vi "运维调试_总磷.vi"() -> ()   [LabVIEW 2016, in "斯坦道总磷.lvlib"]
uses:
  <vilib>/Utility/miscctls.llb/LVPointTypeDef.ctl
  <vilib>/Utility/config.llb/NI_LVConfig.lvlib
  <vilib>/ptbypt/NI_PtbyPt.lvlib
panel:
  in  "远程标样校准":enum16{"标液1", "标液2", "标液3", "标液4"}(ring)
  in  "远程校准量程":enum16{"低量程", "高量程"}(ring)
  out "固件版本号":string
  in  "定时设置":cluster{"启动":bool, "控制命令":T1, "测量参数":T2}(xcontrol)
  out "模块版本号":string
  out "单位:":T3(ring)
  out "运行状态":T4 {"数据时间:" format="%<%y/%m/%d %H:%M:%S>T"; "仪器时间:" format="%<%y/%m/%d %H:%M:%S>T"}
  in  "校准按钮":T5
  out "温度2":sgl
  out "温度1":sgl
  out "ADC":sgl
  out "F3":sgl format="%#.6f"
  out "F2":sgl format="%#.6f"
  out "F1":sgl format="%#.6f"
  out "F0":sgl format="%#.6f"
  out "二级权限":bool
  out "一级权限":bool
  out "输入密码":u32
  out "权限锁":bool
  in  "流程固件":bool
  in  "仪器参数设置":bool
  in  "量程参数读取":T6
  in  "模块启用":bool
  in  "串口设置":bool
  in  "公式一键写入":bool
  in  "流程路径":path=path "C:/Users/STD/Documents/斯坦道流程文件/流程.xml"
  in  "曲线模型":cluster{"X^2":dbl, "X":dbl, "B":dbl, "r^2":dbl}(xcontrol)
  out "字符串":string
  in  "质控参数设置":bool
  in  "数组":string[](array[string])
  in  "量程切换阈值写入":bool
  in  "量程切换阈值读取":bool
  in  "参数下拉列表":enum16{"总磷", "总氮"}(ring)
  in  "量程下拉列表":enum16{"低量程", "高量程"}(ring)
  in  "测量模式下拉列表":enum16{"水样测量", "零点核查", "跨度核查", "标样核查", "加标回收"}(ring)
  in  "公式":cluster{"X^2":dbl, "X":dbl, "b":dbl}
  in  "写公式":bool
  in  "读公式":bool
  in  "返回":bool
  in  "设置":bool
  out "集成报警信息":string
  in  "停止":bool
  in  "手动启动":bool
  in  "单步测试":bool
  out "多列列表框":i32(listbox)
  # "参数设置"
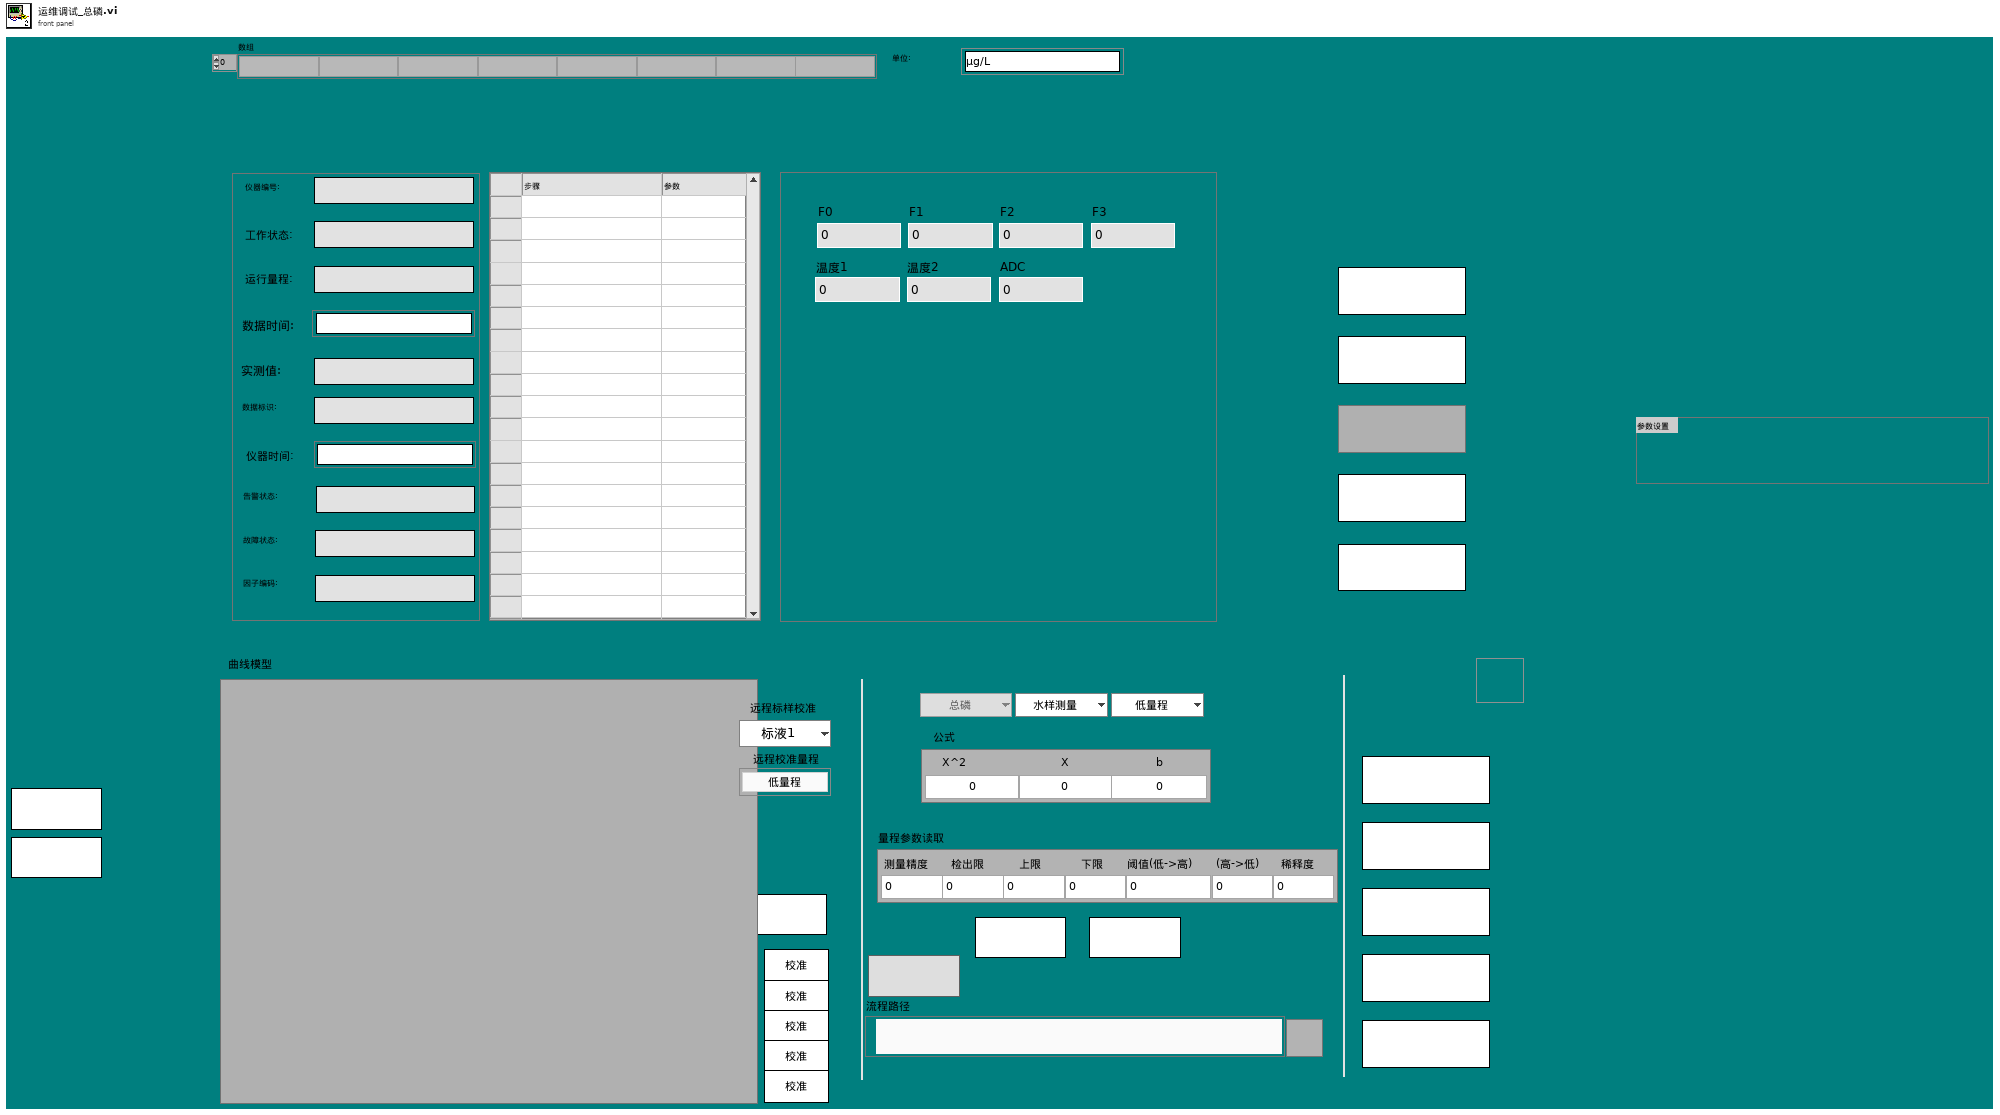
[diagram p1: front panel]
types:
  T1 = typedef "定时设置.xctl/国标控制命令.ctl" = enum16{"启动测量", "标样核查", "零点核查", "跨度核查", "空白测试", "平行样测试", "加标回收", "空白校准", "标样校准", "初始化（清洗）", "停止测试", "仪器重启", "校时", "模式设置", "测量间隔设置"}
  T2 = typedef "定时设置.xctl/测量参数.ctl" = u16
  T3 = enum16{"μg/L", "mg/L", "ppm", "mg/m3", "cm", "ppb", "μg/m3", "%", "nmol/mol", "μmol/mol", "MPN/L", "MPN/100ml", "ng/m3", "NTU", "无量纲", "mS/cm", "μS/cm", "℃", "mV", "cells/L"}
  T4 = cluster{"仪器编号:":string, "工作状态:":string, "运行量程: ":string, "数据时间:":timestamp, "实测值:":string, "数据标识: ":string, "仪器时间:":timestamp, "告警状态: ":string, "故障状态:  ":string, "因子编码:":string}
  T5 = cluster{"校准1":bool, "校准2":bool, "校准3":bool, "校准4":bool, "校准5":bool}
  T6 = cluster{"测量精度":dbl, "检出限":dbl, "上限":dbl, "下限":dbl, "阈值(低->高)":dbl, "(高->低)":dbl, "稀释度":dbl}
  T7 = cluster{"时间源选择":enum16{"系统时间源", "仪器时间源"}, "外部时间源":timestamp}
  T8 = cluster{"系统时间":timestamp, "工作状态":enum16{"空闲", "水样测试", "标样核查", "零点核查", "跨度核查", "空白测试", "平行样测试", "加标回收", "空白校准", "标样校准", "初始化（清洗）"}, "测量模式":enum16{"待机", "连续模式", "周期模式", "定点模式", "受控模式", "手动模式"}, "告警代码":u16, "故障代码":u16, "日志代码":u16, "软件版本":u16, "F0":sgl, "F1":sgl, "F2":sgl, "F3":sgl, "T":sgl, "H":sgl, "id":u16, "flowid":u16, "量程":u16, "总磷控温温度1":sgl, "营养盐控温温度2":sgl, "ADC":sgl}
  T9 = enum32{"Bad", "Idle", "Run top level", "Running"}
  T10 = enum16{"空闲", "水样测试", "标样核查", "零点核查", "跨度核查", "空白测试", "平行样测试", "加标回收", "空白校准", "标样校准", "初始化（清洗）"}
  T11 = typedef "LVPointTypeDef.ctl" = cluster{"Horizontal":i16, "Vertical":i16}
  T12 = cluster{"因子编码":u32, "单位":u16, "标样参考值":sgl, "水样数据时间":timestamp, "水样实测值":sgl, "水样数据标识":string, "标样数据时间":timestamp, "标样实测值":sgl, "标样数据标识":string, "空白数据时间":timestamp, "空白实测值":sgl, "空白数据标识":string, "零点核查数据时间":timestamp, "零点核查实测值":sgl, "零点核查数据标识":string, "跨度核查数据时间":timestamp, "跨度核查实测值":sgl, "跨度核查数据标识":string, "加标回收数据时间":timestamp, "加标回收实测值":sgl, "加标回收数据标识":string, "平行样数据时间":timestamp, "平行样实测值":sgl, "平行样数据标识":string, "F0":sgl, "F1":sgl, "F2":sgl, "F3":sgl, "F4":sgl, "F5":sgl, "F6":sgl, "F7":sgl, "温度":sgl, "湿度":sgl, "X值":sgl, "fidrange":u16}
  T13 = enum16{"待机", "连续模式", "周期模式", "定点模式", "受控模式", "手动模式"}
  T14 = cluster{"Major":u16, "Minor":u16, "Fix":u16, "Build":u16}
  T15 = typedef "NI_LVConfig.lvlib/Config Data RefNum.ctl" = refnum<k1>
  T16 = enum8{"Enabled", "Disabled", "Disabled and Grayed Out"}
  T17 = cluster{"运行模式":enum16{"维护模式", "常规模式", "应急模式", "质控模式"}, "质控频次":enum16{"关闭", "每天", "星期一", "星期二", "星期三", "星期四", "星期五", "星期六", "星期日"}, "空白核查时间":u16, "跨度核查时间":u16, "24H周期设置":bool[]}
  T18 = cluster{"时间标识":timestamp, "设备":string, "日志信息":string, "备注":string}
  T19 = cluster{"参数":string, "报警内容":string, "报警分析":string}
  T20 = cluster{"启动模式":enum16{"跨度核查", "水样测量", "空白核查", "标样核查", "加标回收"}, "启动参数":u16, "量程":enum16{"低量程", "高量程"}}
  T21 = cluster{"时间标识":timestamp, "设备":string, "日志信息":string, "流程参数":string}
  T22 = typedef "LVRowAndColumnUnsignedTypeDef.ctl" = cluster{"Row":u32, "Column":u32}
  T23 = cluster{"参数下拉列表":enum16{"总磷", "总氮"}, "测量模式下拉列表":enum16{"水样测量", "零点核查", "跨度核查", "标样核查", "加标回收"}, "量程下拉列表":enum16{"低量程", "高量程"}}
  T24 = cluster{"站号":u16, "量程切换":enum32{"H", "L", "AUTO"}, "控制命令":enum16{"启动测量", "标样核查", "零点核查", "跨度核查", "空白测试", "平行样测试", "加标回收", "空白校准", "标样校准", "初始化（清洗）", "停止测试", "仪器重启", "校时", "模式设置", "测量间隔设置"}, "模式设置":enum16{"待机", "连续模式", "周期模式", "定点模式", "受控模式", "手动模式"}, "测量间隔":u16}
  T25 = cluster{"水样测试量程模式":enum16{"H", "L", "AUTO"}, "空白核查量程模式":enum16{"H", "L", "AUTO"}, "跨度核查量程模式":enum16{"H", "L", "AUTO"}, "加标回收量程模式":enum16{"H", "L", "AUTO"}}
  T26 = cluster{"总磷跨度值":dbl, "总磷零点标准液浓度":dbl, "总磷跨度标准液浓度":dbl, "总磷标准液标准浓度":dbl}
  T27 = cluster{"确定":bool, "总磷跨度值":dbl, "总磷零点标准液浓度":dbl, "总磷跨度标准液浓度":dbl, "总磷标准液标准浓度":dbl}
  T28 = cluster{"测量量程":dbl, "测量精度":dbl, "测量间隔":dbl, "消解温度":dbl, "消解时长":dbl, "空白校准时间":timestamp, "曲线截距":dbl, "曲线斜率":dbl, "测量检出限":dbl, "测量信号值":dbl, "线性相关系数":dbl, "二次多项式系数":dbl, "标样校准时间":timestamp, "稀释倍数":dbl, "三项式系数":dbl, "空白标定系数":dbl, "量程系数":dbl, "F0/ORPA":dbl, "F1/ORPB":dbl, "F2/ORPK":dbl, "F3":dbl, "F4":dbl, "F5":dbl, "F6":dbl, "F7":dbl, "X0/滴定数":dbl, "量程":dbl}
  T29 = cluster{"确定":bool, "测量量程":dbl, "测量精度":dbl, "测量间隔":dbl, "消解温度":dbl, "消解时长":dbl, "空白校准时间":timestamp, "曲线截距":dbl, "曲线斜率":dbl, "测量检出限":dbl, "测量信号值":dbl, "线性相关系数":dbl, "二次多项式系数":dbl, "标样校准时间":timestamp, "稀释倍数":dbl, "三项式系数":dbl, "空白标定系数":dbl, "量程系数":dbl, "F0/ORPA":dbl, "F1/ORPB":dbl, "F2/ORPK":dbl, "F3":dbl, "F4":dbl, "F5":dbl, "F6":dbl, "F7":dbl, "X0/滴定数":dbl, "量程":dbl}
  T30 = cluster{"标液浓度1":dbl, "标液浓度2":dbl, "标液浓度3":dbl, "标液浓度4":dbl, "标液浓度5":dbl}
  T31 = cluster{"测量精度":u16, "检出限":dbl, "上限":dbl, "下限":dbl, "阈值（低->高）":dbl, "阈值（高->低）":dbl, "稀释度":dbl}
  T32 = enum16{"Left Button", "Center Button", "Right Button", "Window Close"}
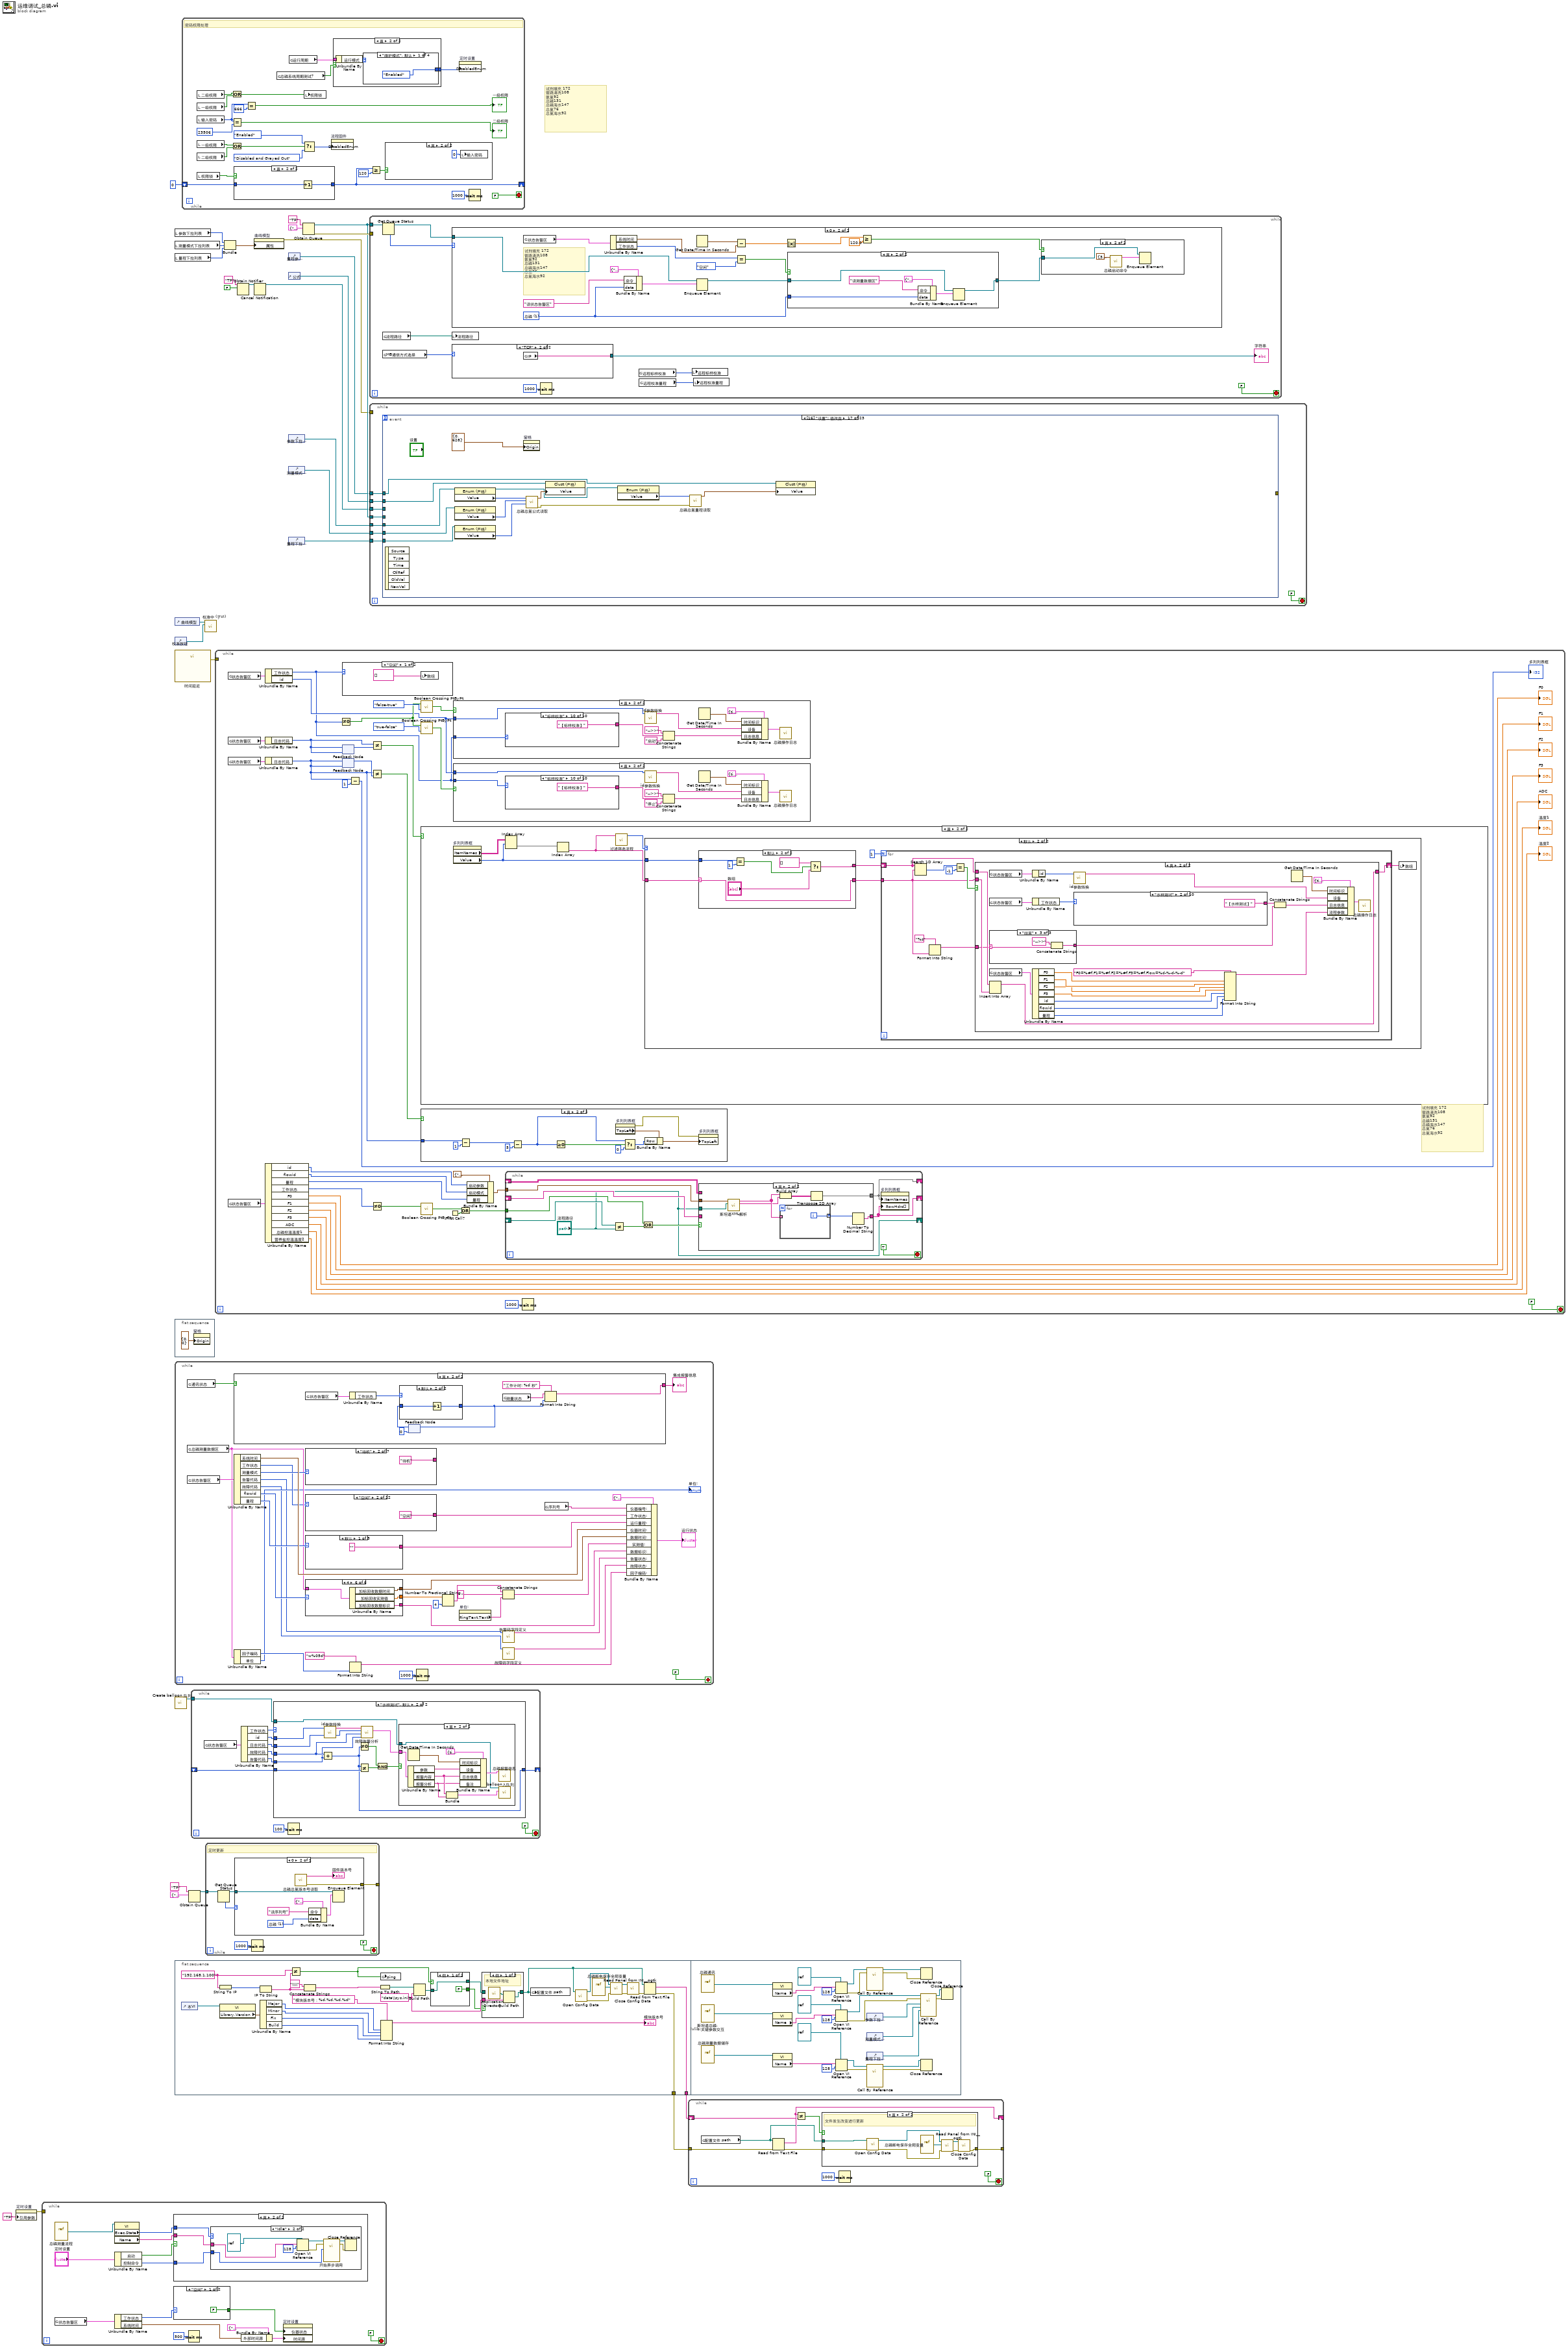
[diagram p0: block diagram]
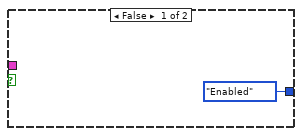
[diagram p5: hidden frame]
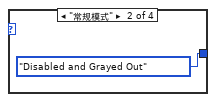
[diagram p6: hidden frame]
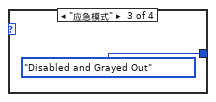
[diagram p7: hidden frame]
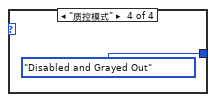
[diagram p8: hidden frame]
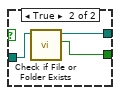
[diagram p11: hidden frame]
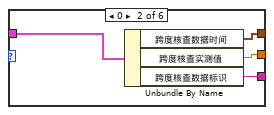
[diagram p15: hidden frame]
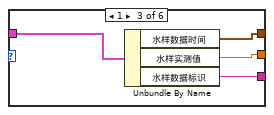
[diagram p16: hidden frame]
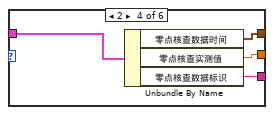
[diagram p17: hidden frame]
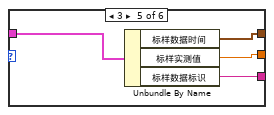
[diagram p18: hidden frame]
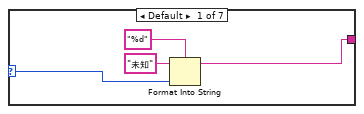
[diagram p19: hidden frame]
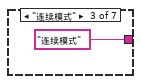
[diagram p20: hidden frame]
diagram:
  # "试剂填充 172 \n管路清洗108\n氨氮92\n总磷131\n总磷海水147\n总氮76\n总氮海水92"
  n1 = property on="定时设置" class="定时设置 (严格)"("引用参数"="TP") -> (error out=w1:errorcluster)  [unwired: 2 in, 1 out]
  n2 = while {
    tunnel: w1 -> [_]
    stop <- FALSE stop-if-true
    n3 = vi-ref "总磷测量流程.vi"() -> (w42:refnum<vi>)
    n4 = global read "VAR总磷全局变量.vi" "状态告警区"() -> (w36:T8)
    n5 = property class="VI"(reference=w42) -> ("Exec.State"=w40:T9, "Name"=w41:string)  [unwired: 1 in, 2 out]
    n6 = Unbundle By Name("定时设置") -> ("启动"=w37:bool, "控制命令"=w38:T1)
    n7 = Unbundle By Name(w36) -> ("工作状态"=w35:T10, "系统时间"=w32:timestamp)
    n8 = case shown="真" w37 {
      tunnel: w41 -> [_ w49]
      tunnel: w38 -> [_ w48]
      tunnel: w40 -> [_ w47]
      frame False {
      }
      frame True {
        n9 = case shown="\"Idle\"" w47 {
          tunnel: w49 -> [_ w53]
          tunnel: w48 -> [_ w51]
          frame "Bad", Default {
          }
          frame "Idle" {
            n10 = Open VI Reference(type specifier VI Refnum (for type only)=refnum<vi> refnum, vi path=w53, options=128 ("选项")) -> (vi reference=w54:refnum<vi>, error out=w55:errorcluster)  [unwired: 3 in]
            n11 = call-by-ref "开始异步调用"(reference=w54, error in=w55, "控制命令"=w51) -> (reference out=w56:refnum<vi>, error out=w57:errorcluster)  [unwired: 11 in]
            n12 = Close Reference(reference=w56, error in (no error)=w57) -> ()  [unwired: 1 out]
          }
        }
      }
    }
    n13 = case shown="\"空闲\"" w35 {
      tunnel: [FALSE TRUE] -> w34
      frame "空闲" {
      }
      frame "水样测试", Default {
      }
    }
    n14 = Wait (ms)(milliseconds to wait=u32 500 ("等待时间（毫秒）")) -> ()  [unwired: 1 out]
    n15 = Bundle By Name(cluster=T7 {"时间源选择"=enum."仪器时间源", "外部时间源"=timestamp(0 s since 1904-01-01)} ("时间源"), "外部时间源"=w32) -> (w31:T7)
    n16 = property on="定时设置" class="定时设置 (严格)"("仪器状态"=w34, "时间源"=w31) -> ()  [unwired: 2 in, 2 out]
  }
  n17 = local read "参数下拉列表"() -> (w11:enum16{"总磷", "总氮"})
  n18 = local read "测量模式下拉列表"() -> (w10:enum16{"水样测量", "零点核查", "跨度核查", "标样核查", "加标回收"})
  n19 = local read "量程下拉列表"() -> (w9:enum16{"低量程", "高量程"})
  n20 = control-ref of="曲线模型"() -> (w5:refnum<vi>)
  n21 = control-ref of="校准按钮"() -> (w6:refnum<vi>)
  n22 = call "时间延迟"() -> ("error out"=w22:errorcluster)  [unwired: 11 in]
  n23 = flat-sequence {
    frame #0 {
      n24 = property on="窗格" class="Pane"("Origin"=T11 {"Horizontal"=0, "Vertical"=0} ("原点")) -> ()  [unwired: 2 in, 2 out]
    }
  }
  n25 = while {
    stop <- FALSE stop-if-true
    n26 = global read "VAR总磷全局变量.vi" "通讯状态"() -> (w88:bool)
    n27 = global read "VAR总磷全局变量.vi" "总磷测量数据区"() -> (w78:T12)
    n28 = global read "VAR总磷全局变量.vi" "状态告警区"() -> (w79:T8)
    n29 = case shown="真" w88 {
      tunnel: ["通讯异常" ("集成报警信息") w141] -> w87
      frame False {
      }
      frame True {
        n30 = global read "VAR总磷全局变量.vi" "状态告警区"() -> (w147:T8)
        n31 = Unbundle By Name(w147) -> ("工作状态"=w146:T10)
        n32 = feedback #1(0) -> (w144:i32)
        n33 = case shown="默认" w146 {
          tunnel: w144 -> [_ w149]
          tunnel: [_ w148] -> w142
          frame "空闲" {
          }
          frame Default {
            n34 = Increment(x=w149) -> (x+1=w148:i32)
          }
        }
        n35 = feedback-in #1(w142) -> ()
        n36 = global read "VAR总磷全局变量.vi" "测量状态"() -> (w140:string)
        n37 = Format Into String(format string="工作计时: %d 秒" ("格式字符串"), initial string=w140, w142) -> (resulting string=w141:string)  [unwired: 1 in, 1 out]
      }
    }
    "集成报警信息" <- w87
    n38 = Unbundle By Name(w79) -> ("系统时间"=w86:timestamp, "工作状态"=w76:T10, "测量模式"=w82:T13, "告警代码"=w62:u16, "故障代码"=w60:u16, "flowid"=w75:u16, "量程"=w84:u16)
    n39 = Unbundle By Name(w78) -> ("因子编码"=w80:u32, "单位"=→"单位:":u16)
    n40 = case shown="\"待机\"" w82 {
      selector: w82 -> [w111 _ _ _ _ _ _]
      tunnel: [w112 "待机" "连续模式" "周期模式" "定点模式" "受控模式" "手动模式"] -> _
      frame Default {
        n41 = Format Into String(format string="%d" ("格式字符串"), initial string="未知" ("工作状态"), w111) -> (resulting string=w112:string)  [unwired: 1 in, 1 out]
      }
      frame "待机" {
      }
      frame "连续模式" {
      }
      frame "周期模式" {
      }
      frame "定点模式" {
      }
      frame "受控模式" {
      }
      frame "手动模式" {
      }
    }
    n42 = case shown="\"空闲\"" w76 {
      selector: w76 -> [w124 _ _ _ _ _ _ _ _ _ _ _]
      tunnel: [w125 "空闲" ("工作状态") "水样测量" ("工作状态") "标样核查" ("工作状态") "零点核查" ("工作状态") "跨度核查" ("工作状态") "空白测试" ("工作状态") "平行样测试" ("工作状态") "加标回收" ("工作状态") "空白校准" ("工作状态") "标样校准" ("工作状态") "初始化" ("工作状态")] -> w85
      frame Default {
        n43 = Format Into String(format string="%d" ("格式字符串"), initial string="未知" ("工作状态"), w124) -> (resulting string=w125:string)  [unwired: 1 in, 1 out]
      }
      frame "空闲" {
      }
      frame "水样测试" {
      }
      frame "标样核查" {
      }
      frame "零点核查" {
      }
      frame "跨度核查" {
      }
      frame "空白测试" {
      }
      frame "平行样测试" {
      }
      frame "加标回收" {
      }
      frame "空白校准" {
      }
      frame "标样校准" {
      }
      frame "初始化（清洗）" {
      }
    }
    n44 = case shown="默认" w84 {
      tunnel: ["" ("字符串") "低量程" ("字符串") "高量程" ("字符串")] -> w83
      frame Default {
      }
      frame 0 {
      }
      frame 1 {
      }
    }
    n45 = case shown="4" w75 {
      tunnel: [_ w94 w98 w102 w106 w110] -> w72
      tunnel: [_ w92 w97 w101 w105 w109] -> w68
      tunnel: [_ w91 w96 w100 w104 w108] -> w64
      tunnel: w78 -> [_ w93 w95 w99 w103 w107]
      frame Default {
      }
      frame 0 {
        n46 = Unbundle By Name(w93) -> ("跨度核查数据时间"=w94:timestamp, "跨度核查实测值"=w92:sgl, "跨度核查数据标识"=w91:string)
      }
      frame 1 {
        n47 = Unbundle By Name(w95) -> ("水样数据时间"=w98:timestamp, "水样实测值"=w97:sgl, "水样数据标识"=w96:string)
      }
      frame 2 {
        n48 = Unbundle By Name(w99) -> ("零点核查数据时间"=w102:timestamp, "零点核查实测值"=w101:sgl, "零点核查数据标识"=w100:string)
      }
      frame 3 {
        n49 = Unbundle By Name(w103) -> ("标样数据时间"=w106:timestamp, "标样实测值"=w105:sgl, "标样数据标识"=w104:string)
      }
      frame 4 {
        n50 = Unbundle By Name(w107) -> ("加标回收数据时间"=w110:timestamp, "加标回收实测值"=w109:sgl, "加标回收数据标识"=w108:string)
      }
    }
    n51 = Format Into String(format string="w%05d" ("格式字符串"), w80) -> (resulting string=w63:string)  [unwired: 2 in, 1 out]
    n52 = Wait (ms)(milliseconds to wait=u32 1000 ("等待时间（毫秒）")) -> ()  [unwired: 1 out]
    n53 = Number To Fractional String(number=w68, precision (6)=i16 4 ("精度(6)")) -> (F-format string=w70:string)  [unwired: 2 in]
    n54 = property on="单位:" class="Enum (严格)"() -> ("RingText.Text"=w66:string)  [unwired: 2 in, 2 out]
    n55 = Concatenate Strings(w70, " " ("字符串"), w66) -> (w65:string)
    n56 = call "告警码字段定义.vi"("告警代码"=w62) -> ("字符串"=w61:string)  [unwired: 8 in, 2 out]
    n57 = call "故障码字段定义.vi"("故障代码"=w60) -> ("字符串"=w59:string)  [unwired: 10 in]
    n58 = global read "VAR总磷全局变量.vi" "序列号"() -> (w77:string)
    n59 = Bundle By Name(cluster=T4 {"仪器编号:"="", "工作状态:"="", "运行量程: "="", "数据时间:"=timestamp(0 s since 1904-01-01), "实测值:"="", "数据标识: "="", "仪器时间:"=timestamp(0 s since 1904-01-01), "告警状态: "="", "故障状态:  "="", "因子编码:"=""} ("运行状态"), "仪器编号:"=w77, "工作状态:"=w85, "运行量程:"=w83, "仪器时间:"=w86, "数据时间:"=w72, "实测值:"=w65, "数据标识:"=w64, "告警状态:"=w61, "故障状态:"=w59, "因子编码:"=w63) -> (→"运行状态":T4)
  }
  n60 = call "Create balloon 队列.vi"() -> ("队列输出"=w3:refnum<queue>)  [unwired: 11 in]
  n61 = flat-sequence {
    tunnel: [w159] -> w4
    tunnel: [w158] -> w7
    frame #0 {
      w172 = "data\\sys.ini" ("名称或相对路径")
      w164 = "192.168.1.100" ("名称")
      n62 = control-ref of="本VI"() -> (w157:refnum<vi>)
      n63 = String To IP(1:w164) -> (0:w171:u32)
      n64 = property class="VI"(reference=w157) -> ("Library.Version"=w156:T14)  [unwired: 1 in, 2 out]
      n65 = IP To String(2:w171) -> (0:w168:string)  [unwired: 1 in]
      n66 = Unbundle By Name(w156) -> ("Major"=w154:u16, "Minor"=w153:u16, "Fix"=w152:u16, "Build"=w151:u16)
      n67 = Not Equal?(x=w164, y=w168) -> (x != y?=w162:bool)
      n68 = Concatenate Strings("\\\\" ("字符串"), w168) -> (w169:string)
      n69 = String To Path(string=w169) -> (path=w163:path)
      n70 = global write "VAR总磷全局变量.vi" "ping"(w162) -> ()
      n71 = Format Into String(format string="模块版本号：%d.%d.%d.%d" ("格式字符串"), w154, w153, w152, w151) -> (resulting string=→"模块版本号":string)  [unwired: 2 in, 1 out]
      n72 = Build Path(base path=w163, name or relative path=w172) -> (appended path=w167:path)
      n73 = case shown="假" w162 {
        tunnel: w167 -> [w178 w182]
        tunnel: [w178 w181] -> w166
        tunnel: [FALSE w180] -> w165
        frame False {
        }
        frame True {
          n74 = call <vilib>:"Check if File or Folder Exists.vi"("path"=w182) -> ("file or folder exists?"=w180:bool, "dup path"=w181:path)  [unwired: 8 in, 1 out]
        }
      }
      n75 = case shown="假" w165 {
        tunnel: w166 -> [_ w186]
        tunnel: [w184 w186] -> w161
        tunnel: w172 -> [w183 _]
        frame False {
          # "本地文件地址"
          n76 = call <vilib>:"Application Directory.vi"() -> ("Application Directory"=w185:path)
          n77 = Build Path(base path=w185, name or relative path=w183) -> (appended path=w184:path)
        }
        frame True {
          # "网络共享地址"
        }
      }
      n78 = global write "VAR总磷全局变量.vi" "配置文件 path"(w161) -> ()
      n79 = call <vilib>:"Open Config Data.vi"("configuration file path"=w161) -> ("error out"=w174:errorcluster, "refnum"=w177:T15)  [unwired: 8 in, 1 out]
      n80 = vi-ref "总磷断电保存全局变量.vi"() -> (w176:refnum<vi>)
      n81 = call <userlib>:"Read Panel from INI__ogtk.vi"("error in (no error)"=w174, "VI ref"=w176, "refnum"=w177) -> ("error out"=w173:errorcluster, "refnum out"=w175:T15)  [unwired: 7 in]
      n82 = call <vilib>:"Close Config Data.vi"("error in (no error)"=w173, "refnum"=w175) -> ("error out"=w160:errorcluster)  [unwired: 8 in, 1 out]
      n83 = Read from Text File(file (use dialog)=w161, error in=w160) -> (text=w158:string, error out=w159:errorcluster)  [unwired: 2 in, 2 out]
    }
    frame #1 {
      n84 = vi-ref "总磷通讯.vi"() -> (w213:refnum<vi>)
      n85 = vi-ref "斯坦道总磷.lvlib:关键参数交互.vi"() -> (w190:refnum<vi>)
      n86 = vi-ref "总磷测量数据储存.vi"() -> (w205:refnum<vi>)
      n87 = property class="VI"(reference=w213) -> ("Name"=w212:string)  [unwired: 1 in, 2 out]
      n88 = property class="VI"(reference=w190) -> ("Name"=w191:string)  [unwired: 1 in, 2 out]
      n89 = property class="VI"(reference=w205) -> ("Name"=w198:string)  [unwired: 1 in, 2 out]
      n90 = Open VI Reference(type specifier VI Refnum (for type only)=refnum<vi> refnum, vi path=w212, options=128 ("选项")) -> (vi reference=w210:refnum<vi>, error out=w208:errorcluster)  [unwired: 3 in]
      n91 = Open VI Reference(type specifier VI Refnum (for type only)=refnum<vi> refnum, vi path=w191, options=128 ("选项")) -> (vi reference=w193:refnum<vi>, error out=w195:errorcluster)  [unwired: 3 in]
      n92 = Open VI Reference(type specifier VI Refnum (for type only)=refnum<vi> refnum, vi path=w198, options=128 ("选项")) -> (vi reference=w200:refnum<vi>, error out=w202:errorcluster)  [unwired: 3 in]
      n93 = call-by-ref "?"(reference=w210, error in=w208) -> (reference out=w206:refnum<vi>, error out=w207:errorcluster)  [unwired: 12 in]
      n94 = control-ref of="参数下拉列表"() -> (w187:refnum<vi>)
      n95 = control-ref of="测量模式下拉列表"() -> (w188:refnum<vi>)
      n96 = control-ref of="量程下拉列表"() -> (w189:refnum<vi>)
      n97 = call-by-ref "?"(reference=w200, error in=w202) -> (reference out=w204:refnum<vi>, error out=w203:errorcluster)  [unwired: 12 in]
      n98 = Close Reference(reference=w206, error in (no error)=w207) -> ()  [unwired: 1 out]
      n99 = call-by-ref "?"(reference=w193, error in=w195, "量程下拉列表"=w189, "测量模式下拉列表"=w188, "测量参数"=w187) -> (reference out=w197:refnum<vi>, error out=w196:errorcluster)  [unwired: 9 in]
      n100 = Close Reference(reference=w204, error in (no error)=w203) -> ()  [unwired: 1 out]
      n101 = Close Reference(reference=w197, error in (no error)=w196) -> ()  [unwired: 1 out]
    }
  }
  n102 = while {
    shift-right: [w219] -> _
    shift-left: u32 0 ("等待时间（毫秒）") -> [w220]
    stop <- FALSE stop-if-true
    # "密码权限处理"
    n103 = local read "二级权限"() -> (w227:bool)
    n104 = local read "一级权限"() -> (w233:bool)
    n105 = local read "输入密码"() -> (w231:u32)
    n106 = local read "一级权限"() -> (w232:bool)
    n107 = local read "二级权限"() -> (w222:bool)
    n108 = local read "权限锁"() -> (w221:bool)
    n109 = Or(x=w227, y=w233) -> (x .or. y?=w228:bool)
    n110 = Equal?(x=w231, y=u32 23506) -> (x = y?=→"二级权限":bool)
    n111 = Or(x=w232, y=w222) -> (x .or. y?=w223:bool)
    n112 = case shown="真" w221 {
      tunnel: w220 -> [_ w248]
      tunnel: [_ w247] -> w219
      frame False {
      }
      frame True {
        n113 = Increment(x=w248) -> (x+1=w247:u32)
      }
    }
    n114 = Equal?(x=w231, y=u32 666) -> (x = y?=→"一级权限":bool)
    n115 = global read "总磷断电保存全局变量.vi" "总磷系统周期测试?"() -> (w215:bool)
    n116 = global read "总磷断电保存全局变量.vi" "运行周期"() -> (w214:T17)
    n117 = Select(t=T16."Enabled" ("禁用"), s=w223, f=T16."Disabled and Grayed Out" ("禁用")) -> (s? t:f=w224:T16)
    n118 = local write "权限锁"(w228) -> ()
    n119 = property on="流程固件" class="Bool"("DisabledEnum"=w224) -> ()  [unwired: 2 in, 2 out]
    n120 = case shown="真" w215 {
      tunnel: w214 -> [_ w241]
      tunnel: [T16."Enabled" ("禁用") w239] -> w216
      frame False {
      }
      frame True {
        n121 = Unbundle By Name(w241) -> ("运行模式"=w240:enum16{"维护模式", "常规模式", "应急模式", "质控模式"})
        n122 = case shown="\"维护模式\", 默认" w240 {
          tunnel: [T16."Enabled" ("禁用") T16."Disabled and Grayed Out" ("禁用") T16."Disabled and Grayed Out" ("禁用") T16."Disabled and Grayed Out" ("禁用")] -> w239
          frame "维护模式", Default {
          }
          frame "常规模式" {
          }
          frame "应急模式" {
          }
          frame "质控模式" {
          }
        }
      }
    }
    n123 = Greater Or Equal?(x=w219, y=u32 120) -> (x >= y?=w217:bool)
    n124 = case shown="真" w217 {
      frame False {
      }
      frame True {
        n125 = local write "输入密码"(u32 0 ("输入密码")) -> ()
      }
    }
    n126 = property on="定时设置" class="定时设置 (严格)"("DisabledEnum"=w216) -> ()  [unwired: 2 in, 2 out]
    n127 = Wait (ms)(milliseconds to wait=u32 1000 ("等待时间（毫秒）")) -> ()  [unwired: 1 out]
  }
  n128 = Obtain Queue(name (unnamed)="TP" ("名称（未命名）"), element data type=cluster{"命令":string, "data":variant} {"命令"="", "data"=variant}) -> (queue out=w19:refnum<queue>)  [unwired: 3 in, 2 out]
  n129 = while {
    tunnel: w3 -> [w255]
    shift-right: [w251] -> _
    shift-left: _ -> [w252]
    stop <- FALSE stop-if-true
    n130 = global read "VAR总磷全局变量.vi" "状态告警区"() -> (w249:T8)
    n131 = Unbundle By Name(w249) -> ("工作状态"=w250:T10, "id"=w257:u16, "日志代码"=w256:u16, "故障代码"=w254:u16, "告警代码"=w253:u16)
    n132 = case shown="\"水样测试\", 默认" w250 {
      tunnel: w257 -> [_ w272]
      tunnel: w256 -> [_ w271]
      tunnel: w255 -> [_ w268]
      tunnel: w254 -> [_ w267]
      tunnel: w253 -> [_ w266]
      tunnel: w252 -> [w260 w265]
      tunnel: [w260 w264] -> w251
      frame "空闲" {
      }
      frame "水样测试", Default {
        n133 = Add(x=w267, y=w266) -> (x+y=w264:u16)
        n134 = call "id参数转换.vi"("id"=w272) -> ("table输出"=w269:string)  [unwired: 10 in]
        n135 = Not Equal To 0?(x=w264) -> (x != 0?=w263:bool)
        n136 = Not Equal?(x=w264, y=w265) -> (x != y?=w262:bool)
        n137 = call "故障告警分析.vi"("告警代码"=w266, "故障代码"=w267, "运行步序"=w271, "参数"=w269) -> ("报警内容"=w270:T19)  [unwired: 6 in, 1 out]
        n138 = And(x=w263, y=w262) -> (x .and. y?=w261:bool)
        n139 = case shown="真" w261 {
          tunnel: w270 -> [_ w281]
          tunnel: w268 -> [_ w273]
          frame False {
          }
          frame True {
            n140 = Get Date/Time In Seconds() -> (seconds since 1Jan1904=w280:timestamp)
            n141 = Unbundle By Name(w281) -> ("参数"=w277:string, "报警内容"=w276:string, "报警分析"=w275:string)
            n142 = Bundle("报警内容"=w276, "报警分析"=w275) -> (w274:cluster{"报警内容":string, "报警分析":string})  [unwired: 1 in]
            n143 = Bundle By Name(cluster=T18 {"时间标识"=timestamp(0 s since 1904-01-01), "设备"="", "日志信息"="", "备注"=""} ("data in"), "时间标识"=w280, "设备"=w277, "日志信息"=w276, "备注"=w275) -> (w279:T18)
            n144 = call "总磷报警信息.vi"("data in"=w279) -> ()  [unwired: 10 in, 1 out]
            n145 = call "balloon入队列.vi"("报警内容"=w274, "队列"=w273) -> ()  [unwired: 9 in, 1 out]
          }
        }
      }
    }
    n146 = Wait (ms)(milliseconds to wait=u32 100) -> ()  [unwired: 1 out]
  }
  n147 = call "校准中 (子VI).vi"("曲线模型"=w5, "校准按钮"=w6) -> ()  [unwired: 9 in]
  n148 = while {
    tunnel: w19 -> [w286]
    tunnel: [w284] -> _
    stop <- FALSE stop-if-true
    # "定时更新"
    n149 = Get Queue Status(queue=w286) -> (queue out=w283:refnum<queue>, # elements in queue=w282:i32)  [unwired: 2 in, 6 out]
    n150 = case shown="0" w282 {
      tunnel: w283 -> [_ w291]
      tunnel: [_ w289] -> w284
      frame Default {
      }
      frame 0 {
        w292 = u16 1 items=["总磷"=1, "氨氮"=3] ("站号")
        n151 = call "总磷总氮版本号读取.vi"() -> ("error out"=w289:errorcluster, "固件版本号"=→"固件版本号":string)  [unwired: 10 in]
        n152 = Bundle By Name(cluster=cluster{"命令":string, "data":variant} {"命令"="", "data"=variant} ("元素"), "命令"="读序列号", "data"=w292) -> (w290:cluster{"命令":string, "data":variant})
        n153 = Enqueue Element(queue=w291, element=w290) -> ()  [unwired: 2 in, 3 out]
      }
    }
    n154 = Wait (ms)(milliseconds to wait=u32 1000 ("等待时间（毫秒）")) -> ()  [unwired: 1 out]
  }
  n155 = while {
    tunnel: w22 -> [_]
    stop <- FALSE stop-if-true
    # "试剂填充 172 \n管路清洗108\n氨氮92\n总磷131\n总磷海水147\n总氮76\n总氮海水92"
    n156 = global read "VAR总磷全局变量.vi" "状态告警区"() -> (w319:T8)
    n157 = global read "VAR总磷全局变量.vi" "状态告警区"() -> (w317:T8)
    n158 = global read "VAR总磷全局变量.vi" "状态告警区"() -> (w321:T8)
    n159 = global read "VAR总磷全局变量.vi" "状态告警区"() -> (w325:T8)
    n160 = Unbundle By Name(w319) -> ("工作状态"=w302:T10, "id"=w303:u16)
    n161 = Unbundle By Name(w317) -> ("日志代码"=w316:u16)
    n162 = Unbundle By Name(w321) -> ("日志代码"=w313:u16)
    n163 = Unbundle By Name(w325) -> ("id"=w322:u16, "flowid"=w324:u16, "量程"=w323:u16, "工作状态"=w310:T10, "F0"=→"F0":sgl, "F1"=→"F1":sgl, "F2"=→"F2":sgl, "F3"=→"F3":sgl, "ADC"=→"ADC":sgl, "总磷控温温度1"=→"温度1":sgl, "营养盐控温温度2"=→"温度2":sgl)
    n164 = Not Equal To 0?(x=w302) -> (x != 0?=w305:bool)
    n165 = case shown="\"空闲\"" w302 {
      frame "空闲" {
        n166 = local write "数组"(string[] [] ("数组")) -> ()
      }
      frame "水样测试", Default {
      }
    }
    n167 = feedback #2(w316) -> (w318:u16)
    n168 = feedback-in #2(w316) -> ()
    n169 = feedback-in #3(w313) -> ()
    n170 = feedback #3(w313) -> (w330:u16)
    n171 = Subtract(x=w313, y=1) -> (x-y=→"多列列表框":i32)
    n172 = Not Equal?(x=w316, y=w318) -> (x != y?=w315:bool)
    n173 = Not Equal?(x=w313, y=w330) -> (x != y?=w329:bool)
    n174 = Not Equal To 0?(x=w310) -> (x != 0?=w327:bool)
    n175 = call <vilib>:"Boolean Crossing PtByPt.vi"("direction"=enum16{"either", "false-true", "true-false"}."false-true", "input"=w305) -> ("crossing"=w307:bool)  [unwired: 1 in]
    n176 = call <vilib>:"Boolean Crossing PtByPt.vi"("direction"=enum16{"either", "false-true", "true-false"}."true-false", "input"=w305) -> ("crossing"=w304:bool)  [unwired: 1 in]
    n177 = case shown="真" w315 {
      frame False {
      }
      frame True {
        n178 = property on="多列列表框" class="MCListbox (严格)"() -> ("ItemNames"=w376:string[][], "Value"=w372:i32)  [unwired: 2 in, 2 out]
        n179 = Index Array(array=w376, index (row)=w372) -> (element=w375:string[])  [unwired: 1 in]
        n180 = Index Array(array=w375) -> (element=w373:string)  [unwired: 1 in]
        n181 = call "过滤筛选流程.vi"("字符串"=w373) -> ("匹配后偏移量"=w374:i32)  [unwired: 10 in]
        n182 = case shown="默认" w374 {
          tunnel: w373 -> [_ w378]
          tunnel: w372 -> [_ w377]
          frame -1 {
          }
          frame Default {
            n183 = case shown="默认" w378 {
              selector: w378 -> [w384 w391]
              tunnel: [w384 w391] -> w380
              tunnel: [string[] [] ("数组") w386] -> w379
              tunnel: w377 -> [_ w390]
              frame "读数" {
              }
              frame Default {
                n184 = Equal?(x=w390, y=1) -> (x = y?=w388:bool)
                n185 = Select(t=string[] [], s=w388, f="数组") -> (s? t:f=w386:string[])
              }
            }
            n186 = for {
              N: 1 -> [_]
              tunnel: w380 -> [w393]
              shift-right: [w392] -> w381
              shift-left: w379 -> [w394]
              n187 = Search 1D Array(1D array=w394, element=w393) -> (index of element=w397:i32)  [unwired: 1 in]
              n188 = Format Into String(format string="%s" ("格式字符串"), w393) -> (resulting string=w398:string)  [unwired: 2 in, 1 out]
              n189 = Equal?(x=w397, y=-1) -> (x = y?=w395:bool)
              n190 = case shown="真" w395 {
                tunnel: w398 -> [_ w408]
                tunnel: w394 -> [w400 w412]
                tunnel: w393 -> [_ w411]
                tunnel: [w400 w410] -> w392
                frame False {
                }
                frame True {
                  n191 = global read "VAR总磷全局变量.vi" "状态告警区"() -> (w425:T8)
                  n192 = global read "VAR总磷全局变量.vi" "状态告警区"() -> (w405:T8)
                  n193 = case shown="\"结束\"" w408 {
                    selector: w408 -> [w435 w438 w441]
                    tunnel: [w435 w437 w440] -> w407
                    frame Default {
                    }
                    frame "初始化" {
                      n194 = Concatenate Strings("-->>" ("字符串"), w438) -> (w437:string)
                    }
                    frame "结束" {
                      n195 = Concatenate Strings("-->>" ("字符串"), w441) -> (w440:string)
                    }
                  }
                  n196 = global read "VAR总磷全局变量.vi" "状态告警区"() -> (w422:T8)
                  n197 = Insert Into Array(array=w412, new element=w411) -> (w410:string[])  [unwired: 1 in]
                  n198 = Unbundle By Name(w425) -> ("id"=w402:u16)
                  n199 = Unbundle By Name(w405) -> ("工作状态"=w404:T10)
                  n200 = Unbundle By Name(w422) -> ("F0"=w419:sgl, "F1"=w418:sgl, "F2"=w417:sgl, "F3"=w416:sgl, "id"=w415:u16, "flowid"=w414:u16, "量程"=w413:u16)
                  n201 = call "id参数转换.vi"("id"=w402) -> ("table输出"=w401:string)  [unwired: 10 in]
                  n202 = case shown="\"水样测试\"" w404 {
                    tunnel: [_ "【水样测试】" ("字符串") "【标样核查】" ("字符串") "【零点核查】" ("字符串") "【跨度核查】" ("字符串") "【空白测试】" ("字符串") "【平行样测试】" ("字符串") "【加标回收】" ("字符串") "【空白校准】" ("字符串") "【标样校准】" ("字符串")] -> w403
                    frame "空闲", Default {
                    }
                    frame "水样测试" {
                    }
                    frame "标样核查" {
                    }
                    frame "零点核查" {
                    }
                    frame "跨度核查" {
                    }
                    frame "空白测试" {
                    }
                    frame "平行样测试" {
                    }
                    frame "加标回收" {
                    }
                    frame "空白校准" {
                    }
                    frame "标样校准" {
                    }
                  }
                  n203 = Format Into String(format string="F0=%#f,F1=%#f,F2=%#f,F3=%#f,Flow=%d-%-d-%-d" ("格式字符串"), w419, w418, w417, w416, w415, w414, w413) -> (resulting string=w420:string)  [unwired: 2 in, 1 out]
                  n204 = Concatenate Strings(w403, w407) -> (w406:string)
                  n205 = Get Date/Time In Seconds() -> (seconds since 1Jan1904=w423:timestamp)
                  n206 = Bundle By Name(cluster=T21 {"时间标识"=timestamp(0 s since 1904-01-01), "设备"="", "日志信息"="", "流程参数"=""} ("data in"), "时间标识"=w423, "设备"=w401, "日志信息"=w406, "流程参数"=w420) -> (w424:T21)
                  n207 = call "总磷操作日志.vi"("data in"=w424) -> ()  [unwired: 11 in]
                }
              }
            }
            n208 = local write "数组"(w381) -> ()
          }
        }
      }
    }
    n209 = case shown="真" w329 {
      tunnel: w313 -> [_ w466]
      frame False {
      }
      frame True {
        n210 = Subtract(x=w466, y=1) -> (x-y=w464:i32)
        n211 = Subtract(x=w464, y=5) -> (x-y=w468:i32)
        n212 = Greater Or Equal To 0?(x=w468) -> (x >= 0?=w467:bool)
        n213 = property on="多列列表框" class="MCListbox (严格)"() -> (error out=w472:errorcluster, "TopLeft"=w473:T22)  [unwired: 2 in, 1 out]
        n214 = Select(t=w468, s=w467, f=0) -> (s? t:f=w469:i32)
        n215 = Bundle By Name(cluster=w473, "Row"=w469) -> (w474:T22)
        n216 = property on="多列列表框" class="MCListbox (严格)"(error in=w472, "TopLeft"=w474) -> ()  [unwired: 1 in, 2 out]
      }
    }
    n217 = call <vilib>:"Boolean Crossing PtByPt.vi"("input"=w327) -> ("crossing"=w309:bool)  [unwired: 2 in]
    n218 = First Call?() -> (First Call?: T/F=w328:bool)
    n219 = case shown="真" w307 {
      tunnel: w302 -> [_ w361]
      tunnel: w303 -> [_ w353]
      frame False {
      }
      frame True {
        n220 = case shown="\"标样校准\"" w361 {
          tunnel: [_ "【水样测试】" ("字符串") "【标样核查】" ("字符串") "【零点核查】" ("字符串") "【跨度核查】" ("字符串") "【空白测试】" ("字符串") "【平行样测试】" ("字符串") "【加标回收】" ("字符串") "【空白校准】" ("字符串") "【标样校准】" ("字符串")] -> w357
          frame "空闲", Default {
          }
          frame "水样测试" {
          }
          frame "标样核查" {
          }
          frame "零点核查" {
          }
          frame "跨度核查" {
          }
          frame "空白测试" {
          }
          frame "平行样测试" {
          }
          frame "加标回收" {
          }
          frame "空白校准" {
          }
          frame "标样校准" {
          }
        }
        n221 = call "id参数转换.vi"("id"=w353) -> ("table输出"=w352:string)  [unwired: 10 in]
        n222 = Concatenate Strings("-->>" ("字符串"), w357, "启动" ("字符串")) -> (w354:string)
        n223 = Get Date/Time In Seconds() -> (seconds since 1Jan1904=w359:timestamp)
        n224 = Bundle By Name(cluster=T21 {"时间标识"=timestamp(0 s since 1904-01-01), "设备"="", "日志信息"="", "流程参数"=""} ("data in"), "时间标识"=w359, "设备"=w352, "日志信息"=w354) -> (w360:T21)
        n225 = call "总磷操作日志.vi"("data in"=w360) -> ()  [unwired: 11 in]
      }
    }
    n226 = case shown="真" w304 {
      tunnel: w302 -> [_ w342]
      tunnel: w303 -> [_ w334]
      frame False {
      }
      frame True {
        n227 = case shown="\"标样校准\"" w342 {
          tunnel: [_ "【水样测试】" ("字符串") "【标样核查】" ("字符串") "【零点核查】" ("字符串") "【跨度核查】" ("字符串") "【空白测试】" ("字符串") "【平行样测试】" ("字符串") "【加标回收】" ("字符串") "【空白校准】" ("字符串") "【标样校准】" ("字符串")] -> w338
          frame "空闲", Default {
          }
          frame "水样测试" {
          }
          frame "标样核查" {
          }
          frame "零点核查" {
          }
          frame "跨度核查" {
          }
          frame "空白测试" {
          }
          frame "平行样测试" {
          }
          frame "加标回收" {
          }
          frame "空白校准" {
          }
          frame "标样校准" {
          }
        }
        n228 = call "id参数转换.vi"("id"=w334) -> ("table输出"=w333:string)  [unwired: 10 in]
        n229 = Concatenate Strings("-->>" ("字符串"), w338, "停止" ("字符串")) -> (w335:string)
        n230 = Get Date/Time In Seconds() -> (seconds since 1Jan1904=w340:timestamp)
        n231 = Bundle By Name(cluster=T21 {"时间标识"=timestamp(0 s since 1904-01-01), "设备"="", "日志信息"="", "流程参数"=""} ("data in"), "时间标识"=w340, "设备"=w333, "日志信息"=w335) -> (w341:T21)
        n232 = call "总磷操作日志.vi"("data in"=w341) -> ()  [unwired: 11 in]
      }
    }
    n233 = Or(x=w309, y=w328) -> (x .or. y?=w326:bool)
    n234 = Bundle By Name(cluster=T20 {"启动模式"=enum."跨度核查", "启动参数"=1, "量程"=enum."低量程"} ("参数簇"), "启动参数"=w322, "启动模式"=w324, "量程"=w323) -> (w320:T20)
    n235 = while {
      tunnel: w326 -> [w452]
      tunnel: w320 -> [w451]
      shift-right: [w446] -> _
      shift-left: _ -> [w448]
      shift-right: [w447] -> _
      shift-left: _ -> [w449]
      shift-right: ["流程路径"] -> _
      shift-left: _ -> [w445]
      stop <- TRUE stop-if-true
      n236 = Not Equal?(x=w445, y="流程路径") -> (x != y?=w443:bool)
      n237 = Or(x=w452, y=w443) -> (x .or. y?=w444:bool)
      n238 = case shown="真" w444 {
        tunnel: [w454 w462] -> w447
        tunnel: [w453 w461] -> w446
        tunnel: w451 -> [_ w456]
        tunnel: w449 -> [w454 _]
        tunnel: w448 -> [w453 _]
        tunnel: "流程路径" -> [_ w455]
        frame False {
        }
        frame True {
          n239 = call "斯坦道XML解析.vi"("添加的路径"=w455, "参数簇"=w456) -> ("步骤时间"=w457:string[], "步骤名"=w459:string[])  [unwired: 8 in]
          n240 = Build Array(w459, w457) -> (w458:string[][])
          n241 = for {
            tunnel: w459 -> [_] mode=indexing
            tunnel: [w463] -> w460 mode=indexing
            i -> [w463]
          }
          n242 = Transpose 2D Array(2D array=w458) -> (transposed array=w461:string[][])
          n243 = Number To Decimal String(number=w460) -> (decimal integer string=w462:string[])  [unwired: 1 in]
        }
      }
      n244 = property on="多列列表框" class="MCListbox (严格)"("ItemNames"=w446, "RowHdrs[]"=w447) -> ()  [unwired: 2 in, 2 out]
    }
    n245 = Wait (ms)(milliseconds to wait=u32 1000 ("等待时间（毫秒）")) -> ()  [unwired: 1 out]
  }
  n246 = Bundle("参数下拉列表"=w11, "测量模式下拉列表"=w10, "量程下拉列表"=w9) -> (w12:T23)  [unwired: 1 in]
  n247 = Obtain Notifier(name (unnamed)="TP" ("名称（未命名）"), notification data type=FALSE) -> (notifier out=w15:refnum<notifier>)  [unwired: 2 in, 2 out]
  n248 = property on="曲线模型" class="曲线模型 (严格)"("属性"=w12) -> (error out=w18:errorcluster)  [unwired: 2 in, 1 out]
  n249 = Cancel Notification(0:w15) -> (8:w14:refnum<notifier>)  [unwired: 1 in, 2 out]
  n250 = control-ref of="量程参数读取"() -> (w13:refnum<vi>)
  n251 = control-ref of="公式"() -> (w23:refnum<vi>)
  n252 = control-ref of="参数下拉列表"() -> (w25:refnum<vi>)
  n253 = control-ref of="测量模式下拉列表"() -> (w24:refnum<vi>)
  n254 = control-ref of="量程下拉列表"() -> (w26:refnum<vi>)
  n255 = Obtain Queue(name (unnamed)="TP" ("名称（未命名）"), element data type=cluster{"命令":string, "data":variant} {"命令"="", "data"=variant}) -> (queue out=w27:refnum<queue>, error out=w28:errorcluster)  [unwired: 3 in, 1 out]
  n256 = while {
    tunnel: w27 -> [w482]
    tunnel: w28 -> [_]
    stop <- FALSE stop-if-true
    n257 = Get Queue Status(queue=w482) -> (queue out=w478:refnum<queue>, # elements in queue=w477:i32)  [unwired: 2 in, 6 out]
    n258 = global read "总磷断电保存全局变量.vi" "流程路径"() -> (w481:path)
    n259 = global read "总磷断电保存全局变量.vi" "MB通信方式选择"() -> (w479:enum16{"串口", "TCP"})
    n260 = case shown="0" w477 {
      tunnel: w478 -> [_ w498]
      frame Default {
      }
      frame 0 {
        w496 = u16 1 items=["总磷"=1, "氨氮"=3] ("站号")
        # "试剂填充 172 \n管路清洗108\n氨氮92\n总磷131\n总磷海水147\n总氮76\n总氮海水92"
        n261 = global read "VAR总磷全局变量.vi" "状态告警区"() -> (w488:T8)
        n262 = Unbundle By Name(w488) -> ("系统时间"=w495:timestamp, "工作状态"=w487:T10)
        n263 = Bundle By Name(cluster=cluster{"命令":string, "data":variant} {"命令"="", "data"=variant} ("元素"), "命令"="读状态告警区", "data"=w496) -> (w500:cluster{"命令":string, "data":variant})
        n264 = Get Date/Time In Seconds() -> (seconds since 1Jan1904=w494:timestamp)
        n265 = Enqueue Element(queue=w498, element=w500) -> (queue out=w497:refnum<queue>)  [unwired: 2 in, 2 out]
        n266 = Subtract(x=w494, y=w495) -> (x-y=w493:dbl)
        n267 = Equal?(x=w487, y=T10."空闲") -> (x = y?=w485:bool)
        n268 = Absolute Value(x=w493) -> (abs(x)=w492:dbl)
        n269 = case shown="真" w485 {
          tunnel: w497 -> [w502 w505]
          tunnel: w496 -> [_ w504]
          tunnel: [w502 w503] -> w489
          frame False {
          }
          frame True {
            n270 = Bundle By Name(cluster=cluster{"命令":string, "data":variant} {"命令"="", "data"=variant} ("元素"), "命令"="读测量数据区", "data"=w504) -> (w507:cluster{"命令":string, "data":variant})
            n271 = Enqueue Element(queue=w505, element=w507) -> (queue out=w503:refnum<queue>)  [unwired: 2 in, 2 out]
          }
        }
        n272 = Greater Or Equal?(x=w492, y=120.0) -> (x >= y?=w490:bool)
        n273 = case shown="真" w490 {
          tunnel: w489 -> [_ w510]
          frame False {
          }
          frame True {
            n274 = call "总磷启动命令.vi"("参数"=T24 {"站号"=3, "量程切换"=enum."AUTO", "控制命令"=enum."校时", "模式设置"=enum."待机", "测量间隔"=0}) -> ("启动命令"=w509:cluster{"命令":string, "data":variant})  [unwired: 10 in]
            n275 = Enqueue Element(queue=w510, element=w509) -> ()  [unwired: 2 in, 3 out]
          }
        }
      }
    }
    n276 = local write "流程路径"(w481) -> ()
    n277 = case shown="\"TCP\"" w479 {
      tunnel: [w512 w513] -> w480
      frame "串口", Default {
        n278 = global read "总磷断电保存全局变量.vi" "VISA Resource"() -> (w512:refnum<visa-resource-name>)
      }
      frame "TCP" {
        n279 = global read "总磷断电保存全局变量.vi" "IP"() -> (w513:string)
      }
    }
    "字符串" <- w480
    n280 = Wait (ms)(milliseconds to wait=u32 1000 ("等待时间（毫秒）")) -> ()  [unwired: 1 out]
    n281 = global read "总磷断电保存全局变量.vi" "远程标样校准"() -> (w476:enum16{"标液1", "标液2", "标液3", "标液4"})
    n282 = global read "总磷断电保存全局变量.vi" "远程校准量程"() -> (w475:enum16{"低量程", "高量程"})
    n283 = local write "远程标样校准"(w476) -> ()
    n284 = local write "远程校准量程"(w475) -> ()
  }
  n285 = while {
    tunnel: w27 -> [w520]
    tunnel: w26 -> [w519]
    tunnel: w25 -> [w518]
    tunnel: w24 -> [w517]
    tunnel: w23 -> [w516]
    tunnel: w13 -> [w515]
    tunnel: w18 -> [_]
    tunnel: w14 -> [w514]
    stop <- FALSE stop-if-true
    n286 = event shown="[16] \"设置\": 值改变" {
      selector: _ -> [_ _ _ _ _ _ _ _ _ _ _ _ _ _ _ _ _ _ _ _ _ _ _]
      dyn-events: _ -> [_ _ _ _ _ _ _ _ _ _ _ _ _ _ _ _ _ _ _ _ _ _ _]
      timeout: _ -> [_ _ _ _ _ _ _ _ _ _ _ _ _ _ _ _ _ _ _ _ _ _ _]
      tunnel: w520 -> [_ _ _ _ w548 _ w564 _ _ _ _ _ w625 _ w643 w679 _ _ _ _ _ _ _]
      tunnel: w519 -> [_ _ _ w526 _ _ _ _ _ _ _ _ _ _ _ _ w685 _ _ w708 w711 _ _]
      tunnel: w518 -> [_ _ _ w528 _ _ _ _ _ _ _ _ _ _ _ _ w687 _ _ w706 w713 w769 w776]
      tunnel: w517 -> [_ _ _ w527 _ _ _ _ _ _ _ _ _ _ _ _ w686 _ _ w707 w712 _ _]
      tunnel: w516 -> [_ _ _ w529 _ _ _ _ _ _ _ _ _ _ _ _ w688 _ _ w702 _ _ _]
      tunnel: w515 -> [_ _ _ _ _ _ _ _ _ _ _ _ _ _ _ _ w682 _ _ _ _ w767 _]
      tunnel: w514 -> [_ _ _ _ _ _ _ _ _ _ _ _ _ _ _ w674 _ _ _ _ _ _ _]
      tunnel: [_ _ _ w534 _ _ _ _ _ _ _ _ _ _ _ _ _ _ _ _ _ _ _] -> _
      event Timeout {
        n287 = event-data() -> ()  [unwired: 1 in, 3 out]
      }
      event "权限锁": Mouse Down {
        n288 = event-data() -> ("CtlRef"=w523:refnum<vi>)  [unwired: 1 in, 5 out]
        n289 = property class="Bool (严格)"(reference=w523) -> ("Value"=w522:bool)  [unwired: 1 in, 2 out]
        n290 = case shown="真" w522 {
          frame False {
            n291 = call "密码键盘.vi"() -> ("NewNumber"=→"输入密码":dbl)  [unwired: 1 in]
          }
          frame True {
            n292 = local write "输入密码"(u32 0 ("输入密码")) -> ()
          }
        }
      }
      event "流程固件": Value Change {
        n293 = event-data() -> ()  [unwired: 1 in, 6 out]
        n294 = call "流程固件设置对话框.vi"() -> ()  [unwired: 12 in]
      }
      event "测量模式下拉列表", "量程下拉列表", "参数下拉列表": Value Change {
        n295 = event-data() -> ()  [unwired: 1 in, 6 out]
        n296 = property class="Enum (严格)"(reference=w528) -> ("Value"=w533:enum16{"总磷", "总氮"})  [unwired: 1 in, 2 out]
        n297 = property class="Enum (严格)"(reference=w527) -> ("Value"=w532:enum16{"水样测量", "零点核查", "跨度核查", "标样核查", "加标回收"})  [unwired: 1 in, 2 out]
        n298 = property class="Enum (严格)"(reference=w526) -> ("Value"=w531:enum16{"低量程", "高量程"})  [unwired: 1 in, 2 out]
        n299 = call "总磷总氮公式读取.vi"("量程"=w531, "测量模式"=w532, "测量参数"=w533) -> ("公式"=w530:cluster{"X^2":dbl, "X":dbl, "b":dbl})  [unwired: 7 in, 1 out]
        n300 = property class="Clust (严格)"(reference=w529, "Value"=w530) -> ()  [unwired: 1 in, 2 out]
        n301 = local read "参数下拉列表"() -> (w536:enum16{"总磷", "总氮"})
        n302 = local read "测量模式下拉列表"() -> (w537:enum16{"水样测量", "零点核查", "跨度核查", "标样核查", "加标回收"})
        n303 = local read "量程下拉列表"() -> (w538:enum16{"低量程", "高量程"})
        n304 = Bundle("参数下拉列表"=w536, "测量模式下拉列表"=w537, "量程下拉列表"=w538) -> (w535:T23)  [unwired: 1 in]
        n305 = property on="曲线模型" class="曲线模型 (严格)"("属性"=w535) -> (error out=w534:errorcluster)  [unwired: 2 in, 1 out]
      }
      event "串口设置": Value Change {
        n306 = event-data() -> ()  [unwired: 1 in, 6 out]
        n307 = global read "总磷断电保存全局变量.vi" "VISA Resource"() -> (w545:refnum<visa-resource-name>)
        n308 = global read "总磷断电保存全局变量.vi" "MB通信方式选择"() -> (w539:enum16{"串口", "TCP"})
        n309 = global read "总磷断电保存全局变量.vi" "IP"() -> (w544:string)
        n310 = global read "总磷断电保存全局变量.vi" "PORT"() -> (w543:string)
        n311 = call "串口配置.vi"("PORT"=w543, "IP"=w544, "MB通信方式选择"=w539, "请选择串口:"=w545) -> ("PORT 2"=w541:string, "IP 2"=w542:string, "确认 2"=w546:bool, "VISA资源名称 2"=w547:refnum<visa-resource-name>, "MB通信方式选择 2"=w540:enum16{"串口", "TCP"})  [unwired: 3 in]
        n312 = case shown="真" w546 {
          tunnel: w547 -> [_ w553]
          tunnel: w548 -> [_ w552]
          tunnel: w542 -> [_ w551]
          tunnel: w541 -> [_ w550]
          tunnel: w540 -> [_ w549]
          frame False {
          }
          frame True {
            n313 = flat-sequence {
              tunnel: w553 -> [w558]
              tunnel: w552 -> [w559]
              tunnel: w551 -> [w557]
              tunnel: w550 -> [w556]
              tunnel: w549 -> [w555]
              frame #0 {
                n314 = global write "总磷断电保存全局变量.vi" "IP"(w557) -> ()
                n315 = global write "总磷断电保存全局变量.vi" "PORT"(w556) -> ()
                n316 = global write "总磷断电保存全局变量.vi" "MB通信方式选择"(w555) -> ()
                n317 = global write "总磷断电保存全局变量.vi" "VISA Resource"(w558) -> ()
                n318 = Flush Queue(queue=w559) -> (queue out=w554:refnum<queue>)  [unwired: 1 in, 2 out]
                n319 = Enqueue Element(queue=w554, element=cluster{"命令":string, "data":variant} {"命令"="启用模块", "data"=variant} ("元素")) -> ()  [unwired: 2 in, 3 out]
              }
              frame #1 {
                n320 = call "配置文件保存.vi"() -> ()  [unwired: 12 in]
              }
            }
          }
        }
      }
      event "远程校准量程", "远程标样校准": Value Change {
        n321 = event-data() -> ()  [unwired: 1 in, 6 out]
        n322 = flat-sequence {
          frame #0 {
            n323 = global write "总磷断电保存全局变量.vi" "远程标样校准"("远程标样校准") -> ()
            n324 = global write "总磷断电保存全局变量.vi" "远程校准量程"("远程校准量程") -> ()
          }
          frame #1 {
            n325 = call "配置文件保存.vi"() -> ()  [unwired: 12 in]
          }
        }
      }
      event "模块启用": Value Change {
        n326 = event-data() -> ("OldVal"=w565:bool)  [unwired: 1 in, 5 out]
        n327 = Flush Queue(queue=w564) -> (queue out=w563:refnum<queue>)  [unwired: 1 in, 2 out]
        n328 = case shown="假" w565 {
          tunnel: w563 -> [w566 w568]
          frame False {
            n329 = Enqueue Element(queue=w566, element=cluster{"命令":string, "data":variant} {"命令"="停用模块", "data"=variant} ("元素")) -> ()  [unwired: 2 in, 3 out]
          }
          frame True {
            n330 = Enqueue Element(queue=w568, element=cluster{"命令":string, "data":variant} {"命令"="启用模块", "data"=variant} ("元素")) -> ()  [unwired: 2 in, 3 out]
          }
        }
      }
      event "流程路径": Value Change {
        n331 = event-data() -> ()  [unwired: 1 in, 6 out]
        n332 = flat-sequence {
          frame #0 {
            n333 = local read "流程路径"() -> (w570:path)
            n334 = global write "总磷断电保存全局变量.vi" "流程路径"(w570) -> ()
          }
          frame #1 {
            n335 = call "配置文件保存.vi"() -> ()  [unwired: 12 in]
          }
        }
      }
      event "公式一键写入": Value Change {
        n336 = event-data() -> ()  [unwired: 1 in, 6 out]
        n337 = local read "公式"() -> (w571:cluster{"X^2":dbl, "X":dbl, "b":dbl})
        n338 = call "公式复合写入.vi"("公式"=w571) -> ()  [unwired: 11 in]
      }
      event "曲线模型": Value Change {
        n339 = event-data() -> ()  [unwired: 1 in, 6 out]
        n340 = disable-structure shown="禁用" {
          frame Disabled {
            n341 = Unbundle By Name("曲线模型") -> ("X^2"=w574:dbl, "X"=w575:dbl, "B"=w576:dbl)
            n342 = Build Array(w574, w575, w576) -> (w573:dbl[])
            n343 = Array To Cluster(array=w573) -> (cluster=w572:cluster{"[0]":dbl, "[1]":dbl, "[2]":dbl})
            n344 = local write "公式"(w572) -> ()
          }
          frame Enabled {
          }
        }
      }
      event "质控参数设置": Value Change {
        n345 = event-data() -> ()  [unwired: 1 in, 6 out]
        n346 = global read "总磷断电保存全局变量.vi" "总磷自动测试量程配置"() -> (w579:T25)
        n347 = global read "总磷断电保存全局变量.vi" "质控参数设置"() -> (w580:T26)
        n348 = call "总磷质控参数设置.vi"("自动测试量程配置"=w579, "质控参数设置"=w580) -> ("自动测试量程配置输出"=w578:T25, "输出簇"=w581:T27)  [unwired: 8 in]
        n349 = Unbundle By Name(w581) -> ("确定"=w582:bool)
        n350 = case shown="真" w582 {
          tunnel: w581 -> [_ w585]
          tunnel: w580 -> [_ w584]
          tunnel: w578 -> [_ w583]
          frame False {
          }
          frame True {
            n351 = flat-sequence {
              tunnel: w585 -> [w593]
              tunnel: w584 -> [w592]
              tunnel: w583 -> [w586]
              frame #0 {
                n352 = Unbundle By Name(w593) -> ("总磷跨度值"=w591:dbl, "总磷零点标准液浓度"=w590:dbl, "总磷跨度标准液浓度"=w589:dbl, "总磷标准液标准浓度"=w588:dbl)
                n353 = global write "总磷断电保存全局变量.vi" "总磷自动测试量程配置"(w586) -> ()
                n354 = Bundle By Name(cluster=w592, "总磷跨度值"=w591, "总磷零点标准液浓度"=w590, "总磷跨度标准液浓度"=w589, "总磷标准液标准浓度"=w588) -> (w587:T26)
                n355 = global write "总磷断电保存全局变量.vi" "质控参数设置"(w587) -> ()
              }
              frame #1 {
                n356 = call "配置文件保存.vi"() -> ()  [unwired: 12 in]
              }
            }
          }
        }
      }
      event "仪器参数设置": Value Change {
        n357 = event-data() -> ()  [unwired: 1 in, 6 out]
        n358 = global read "总磷断电保存全局变量.vi" "总磷仪器参数"() -> (w595:T28)
        n359 = call "仪器参数设置.vi"("氨氮仪器参数"=w595) -> ("仪器参数设置输出"=w594:T29)  [unwired: 10 in]
        n360 = Unbundle By Name(w594) -> ("确定"=w596:bool)
        n361 = case shown="真" w596 {
          tunnel: w594 -> [_ w598]
          tunnel: w595 -> [_ w597]
          frame False {
          }
          frame True {
            n362 = flat-sequence {
              tunnel: w598 -> [w615]
              tunnel: w597 -> [w614]
              frame #0 {
                n363 = Unbundle By Name(w615) -> ("测量量程"=w613:dbl, "测量精度"=w612:dbl, "测量间隔"=w611:dbl, "消解温度"=w610:dbl, "消解时长"=w608:dbl, "空白校准时间"=w607:timestamp, "曲线截距"=w606:dbl, "曲线斜率"=w605:dbl, "测量检出限"=w604:dbl, "测量信号值"=w603:dbl, "线性相关系数"=w602:dbl, "二次多项式系数"=w601:dbl, "标样校准时间"=w600:timestamp, "稀释倍数"=w599:dbl)
                n364 = Bundle By Name(cluster=w614, "测量量程"=w613, "测量精度"=w612, "测量间隔"=w611, "消解温度"=w610, "消解时长"=w608, "空白校准时间"=w607, "曲线截距"=w606, "曲线斜率"=w605, "测量检出限"=w604, "测量信号值"=w603, "线性相关系数"=w602, "二次多项式系数"=w601, "标样校准时间"=w600, "稀释倍数"=w599) -> (w609:T28)
                n365 = global write "总磷断电保存全局变量.vi" "总磷仪器参数"(w609) -> ()
              }
              frame #1 {
                n366 = call "配置文件保存.vi"() -> ()  [unwired: 12 in]
              }
            }
          }
        }
      }
      event "手动启动": Value Change {
        n367 = event-data() -> ()  [unwired: 1 in, 6 out]
        n368 = call "总磷启动参数对话框.vi"() -> ("标样浓度输出"=w617:dbl, "确认"=w624:bool, "元素"=w618:cluster{"命令":string, "data":variant})  [unwired: 9 in]
        n369 = case shown="真" w624 {
          tunnel: w625 -> [_ w640]
          tunnel: w618 -> [_ w639]
          frame False {
          }
          frame True {
            n370 = Enqueue Element(queue=w640, element=w639) -> ()  [unwired: 2 in, 3 out]
          }
        }
        n371 = Unbundle By Name(w618) -> ("data"=w622:variant)
        n372 = Variant To Data(type=cluster{"站号":u16, "控制命令":u16[]} {"站号"=0, "控制命令"=[]} ("输出簇"), Variant=w622) -> (data=w621:cluster{"站号":u16, "控制命令":u16[]})  [unwired: 1 in, 1 out]
        n373 = Unbundle By Name(w621) -> ("控制命令"=w620:u16[])
        n374 = Index Array(array=w620) -> (element=w619:u16)  [unwired: 1 in]
        n375 = Swap Bytes(anything=w619) -> (byte swapped=w616:u16)
        n376 = case shown="9" w616 {
          tunnel: w617 -> [_ w626 _ _]
          frame 0, Default {
          }
          frame 2 {
            n377 = flat-sequence {
              tunnel: w626 -> [w627]
              frame #0 {
                n378 = global read "总磷断电保存全局变量.vi" "质控参数设置"() -> (w628:T26)
                n379 = Bundle By Name(cluster=w628, "总磷标准液标准浓度"=w627) -> (w629:T26)
                n380 = global write "总磷断电保存全局变量.vi" "质控参数设置"(w629) -> ()
              }
              frame #1 {
                n381 = call "配置文件保存.vi"() -> ()  [unwired: 12 in]
              }
            }
          }
          frame 8 {
            # "空白校准"
            n382 = property on="校准1" class="Bool (严格)"("Val(Sgnl)"=TRUE ("值(信号)")) -> ()  [unwired: 2 in, 2 out]
            n383 = property on="量程下拉列表" class="Enum (严格)"("Val(Sgnl)"=enum16{"低量程", "高量程"}."低量程" ("值(信号)")) -> ()  [unwired: 2 in, 2 out]
          }
          frame 9 {
            # "标样校准"
            n384 = local read "远程标样校准"() -> (w634:enum16{"标液1", "标液2", "标液3", "标液4"})
            n385 = case shown="\"标液4\"" w634 {
              tunnel: TRUE -> [w635 w636 w637 w638]
              frame "标液1", Default {
                n386 = property on="校准2" class="Bool (严格)"("Val(Sgnl)"=w635) -> ()  [unwired: 2 in, 2 out]
              }
              frame "标液2" {
                n387 = property on="校准3" class="Bool (严格)"("Val(Sgnl)"=w636) -> ()  [unwired: 2 in, 2 out]
              }
              frame "标液3" {
                n388 = property on="校准4" class="Bool (严格)"("Val(Sgnl)"=w637) -> ()  [unwired: 2 in, 2 out]
              }
              frame "标液4" {
                n389 = property on="校准5" class="Bool (严格)"("Val(Sgnl)"=w638) -> ()  [unwired: 2 in, 2 out]
              }
            }
            n390 = local read "远程校准量程"() -> (w632:enum16{"低量程", "高量程"})
            n391 = property on="量程下拉列表" class="Enum (严格)"("Val(Sgnl)"=w632) -> ()  [unwired: 2 in, 2 out]
          }
        }
      }
      event "单步测试": Value Change {
        n392 = event-data() -> ()  [unwired: 1 in, 6 out]
        n393 = call "总磷单步调试对话框.vi"() -> ()  [unwired: 12 in]
      }
      event "校准按钮.校准1", "校准按钮.校准2", "校准按钮.校准3", "校准按钮.校准4", "校准按钮.校准5": Value Change {
        n394 = event-data() -> ("CtlRef"=w651:refnum<vi>)  [unwired: 1 in, 5 out]
        n395 = property class="Bool (严格)"(reference=w651) -> ("Label.Text"=w652:string)  [unwired: 1 in, 2 out]
        n396 = property on="曲线模型" class="曲线模型 (严格)"() -> ("浓度属性"=w650:T30)  [unwired: 2 in, 2 out]
        n397 = case shown="\"校准1\", 默认" w652 {
          tunnel: [w658 w661 w664 w667 w670] -> w645
          tunnel: [u16 1 ("校准点1-5") u16 2 ("校准点1-5") u16 3 ("校准点1-5") u16 4 ("校准点1-5") u16 5 ("校准点1-5")] -> w647
          tunnel: w650 -> [w659 w662 w665 w668 w671]
          frame "校准1", Default {
            n398 = Unbundle By Name(w659) -> ("标液浓度1"=w658:dbl)
          }
          frame "校准2" {
            n399 = Unbundle By Name(w662) -> ("标液浓度2"=w661:dbl)
          }
          frame "校准3" {
            n400 = Unbundle By Name(w665) -> ("标液浓度3"=w664:dbl)
          }
          frame "校准4" {
            n401 = Unbundle By Name(w668) -> ("标液浓度4"=w667:dbl)
          }
          frame "校准5" {
            n402 = Unbundle By Name(w671) -> ("标液浓度5"=w670:dbl)
          }
        }
        n403 = Not Equal To 0?(x=w645) -> (x != 0?=w644:bool)
        n404 = Bundle By Name(cluster=cluster{"校准？":bool, "校准点1-5":u16, "校准浓度":dbl} {"校准？"=FALSE, "校准点1-5"=0, "校准浓度"=0.0} ("校准输出"), "校准？"=TRUE, "校准点1-5"=w647, "校准浓度"=w645) -> (w646:cluster{"校准？":bool, "校准点1-5":u16, "校准浓度":dbl})
        n405 = global write "总磷断电保存全局变量.vi" "校准输出"(w646) -> ()
        n406 = local read "量程下拉列表"() -> (w641:enum16{"低量程", "高量程"})
        n407 = case shown="假" w644 {
          tunnel: [cluster{"命令":string, "data":variant} {"命令"="启动", "data"=variant(cluster{"站号":u16, "控制命令":u16[]} {"站号"=1, "控制命令"=[2048, 256]})} ("元素") w654] -> w642
          tunnel: w641 -> [_ w655]
          frame False {
            # "校零"
          }
          frame True {
            # "校标"
            n408 = case shown="\"高量程\"" w655 {
              tunnel: [cluster{"命令":string, "data":variant} {"命令"="启动", "data"=variant(cluster{"站号":u16, "控制命令":u16[]} {"站号"=1, "控制命令"=[2304, 256]})} ("元素") cluster{"命令":string, "data":variant} {"命令"="启动", "data"=variant(cluster{"站号":u16, "控制命令":u16[]} {"站号"=1, "控制命令"=[2304, 257]})} ("元素")] -> w654
              frame "低量程", Default {
              }
              frame "高量程" {
              }
            }
          }
        }
        n409 = Enqueue Element(queue=w643, element=w642) -> ()  [unwired: 2 in, 3 out]
      }
      event "停止": Value Change {
        n410 = event-data() -> ()  [unwired: 1 in, 6 out]
        n411 = Cancel Notification(0:w674) -> (8:w675:refnum<notifier>)  [unwired: 1 in, 2 out]
        n412 = Enqueue Element(queue=w679, element=cluster{"命令":string, "data":variant} {"命令"="启动", "data"=variant(cluster{"站号":u16, "控制命令输出":u16[]} {"站号"=1, "控制命令输出"=[2816]})} ("元素")) -> (queue out=w676:refnum<queue>)  [unwired: 2 in, 2 out]
        n413 = Send Notification(notification=TRUE ("通知"), notifier=w675) -> ()  [unwired: 1 in, 2 out]
        n414 = Enqueue Element(queue=w676, element=cluster{"命令":string, "data":variant} {"命令"="启动", "data"=variant(cluster{"站号":u16, "控制命令输出":u16[]} {"站号"=2, "控制命令输出"=[2816]})} ("元素")) -> ()  [unwired: 2 in, 3 out]
      }
      event "设置": Value Change {
        n415 = event-data() -> ()  [unwired: 1 in, 6 out]
        n416 = property class="Enum (严格)"(reference=w687) -> (reference out=w681:refnum<vi>, "Value"=w692:enum16{"总磷", "总氮"})  [unwired: 1 in, 1 out]
        n417 = property class="Enum (严格)"(reference=w686) -> ("Value"=w691:enum16{"水样测量", "零点核查", "跨度核查", "标样核查", "加标回收"})  [unwired: 1 in, 2 out]
        n418 = property class="Enum (严格)"(reference=w685) -> ("Value"=w690:enum16{"低量程", "高量程"})  [unwired: 1 in, 2 out]
        n419 = property on="窗格" class="Pane"("Origin"=T11 {"Horizontal"=0, "Vertical"=628} ("原点")) -> ()  [unwired: 2 in, 2 out]
        n420 = call "总磷总氮公式读取.vi"("量程"=w690, "测量模式"=w691, "测量参数"=w692) -> ("error out"=w680:errorcluster, "公式"=w689:cluster{"X^2":dbl, "X":dbl, "b":dbl})  [unwired: 7 in]
        n421 = property class="Clust (严格)"(reference=w688, "Value"=w689) -> ()  [unwired: 1 in, 2 out]
        n422 = property class="Enum (严格)"(reference=w681) -> ("Value"=w684:enum16{"总磷", "总氮"})  [unwired: 1 in, 2 out]
        n423 = call "总磷总氮量程读取.vi"("error in (no error)"=w680, "测量参数"=w684) -> ("量程参数读取"=w683:T31)  [unwired: 8 in, 1 out]
        n424 = property class="Clust (严格)"(reference=w682, "Value"=w683) -> ()  [unwired: 1 in, 2 out]
      }
      event "返回": Value Change {
        n425 = event-data() -> ()  [unwired: 1 in, 6 out]
        n426 = property on="窗格" class="Pane"("Origin"=T11 {"Horizontal"=0, "Vertical"=0} ("原点")) -> ()  [unwired: 2 in, 2 out]
      }
      event "公式.X^2", "公式.X", "公式.b", "量程参数读取.测量精度", "量程参数读取.检出限", "量程参数读取.上限", "量程参数读取.下限", "量程参数读取.阈值(低->高)", "量程参数读取.(高->低)", "量程参数读取.稀释度": Mouse Down {
        n427 = event-data() -> ("CtlRef"=w698:refnum<vi>)  [unwired: 1 in, 5 out]
        n428 = property class="DigNum (严格)"(reference=w698) -> (reference out=w696:refnum<vi>, "Value"=w697:dbl)  [unwired: 1 in, 1 out]
        n429 = call "数字键盘.vi"("OldNumber"=w697) -> ("NewNumber"=w695:dbl)
        n430 = property class="DigNum (严格)"(reference=w696, "Val(Sgnl)"=w695) -> ()  [unwired: 1 in, 2 out]
      }
      event "读公式": Value Change {
        n431 = event-data() -> ()  [unwired: 1 in, 6 out]
        n432 = property class="Enum (严格)"(reference=w706) -> ("Value"=w705:enum16{"总磷", "总氮"})  [unwired: 1 in, 2 out]
        n433 = property class="Enum (严格)"(reference=w707) -> ("Value"=w704:enum16{"水样测量", "零点核查", "跨度核查", "标样核查", "加标回收"})  [unwired: 1 in, 2 out]
        n434 = property class="Enum (严格)"(reference=w708) -> ("Value"=w703:enum16{"低量程", "高量程"})  [unwired: 1 in, 2 out]
        n435 = call "总磷总氮公式读取.vi"("量程"=w703, "测量模式"=w704, "测量参数"=w705) -> ("error out"=w700:errorcluster, "公式"=w701:cluster{"X^2":dbl, "X":dbl, "b":dbl})  [unwired: 7 in]
        n436 = property class="Clust (严格)"(reference=w702, "Value"=w701) -> ()  [unwired: 1 in, 2 out]
        n437 = case shown="错误" w700 {
          tunnel: ["读取成功" ("消息") "读取失败" ("消息")] -> w699
          frame No Error {
          }
          frame Error {
          }
        }
        n438 = One Button Dialog(message=w699) -> ()  [unwired: 1 in, 1 out]
      }
      event "写公式": Value Change {
        n439 = event-data() -> ()  [unwired: 1 in, 6 out]
        n440 = call <vilib>:"Three Button Dialog.vi"("Allow user to close window? (TRUE)"=FALSE, "Center Button Text (\"No\")"="一键写入所有公式" ("F按钮名称（“取消”）"), "Left Button Text (\"Yes\")"="写入当前公式" ("T按钮名称（“确定”）"), "message"="即将将左侧拟合公式写入仪器\n请选择写入当前模式还是一键写入所有模式！" ("消息")) -> ("Which Button?"=w714:T32)  [unwired: 7 in]
        n441 = case shown="\"Left Button\", 默认" w714 {
          tunnel: w713 -> [w724 w757 _ _]
          tunnel: w712 -> [w723 w755 _ _]
          tunnel: w711 -> [w722 w756 _ _]
          frame "Left Button", Default {
            n442 = local read "曲线模型"() -> (w730:cluster{"X^2":dbl, "X":dbl, "B":dbl, "r^2":dbl})
            n443 = Unbundle By Name(w730) -> ("X^2"=w729:dbl, "X"=w727:dbl, "B"=w728:dbl)
            n444 = Build Array(w729, w727, w728) -> (w726:dbl[])
            n445 = Array To Cluster(array=w726) -> (cluster=w725:cluster{"[0]":dbl, "[1]":dbl, "[2]":dbl})
            n446 = call "总磷总氮公式写入.vi"("公式"=w725, "量程"="量程下拉列表", "测量模式"="测量模式下拉列表", "测量参数"="参数下拉列表") -> ("error out"=w734:errorcluster)  [unwired: 7 in]
            n447 = local write "公式"(w725) -> ()
            n448 = case shown="无错误" w734 {
              tunnel: ["写入成功" ("消息") "写入失败" ("消息")] -> w735
              tunnel: "测量模式下拉列表" -> [w739 _]
              tunnel: "量程下拉列表" -> [w738 _]
              tunnel: w725 -> [w736 _]
              frame No Error {
                n449 = Equal?(x=w739, y=enum16{"水样测量", "零点核查", "跨度核查", "标样核查", "加标回收"}."水样测量") -> (x = y?=w741:bool)
                n450 = Equal?(x=w738, y=enum16{"低量程", "高量程"}."低量程") -> (x = y?=w740:bool)
                n451 = Compound Arithmetic op=AND ("复合运算")(w741, w740) -> (w737:bool)
                n452 = case shown="真" w737 {
                  tunnel: w736 -> [_ w745]
                  frame False {
                  }
                  frame True {
                    n453 = Unbundle By Name(w745) -> ("[0]"=w748:dbl, "[1]"=w750:dbl, "[2]"=w749:dbl)
                    n454 = global read "总磷断电保存全局变量.vi" "总磷仪器参数"() -> (w747:T28)
                    n455 = Bundle By Name(cluster=w747, "曲线截距"=w749, "曲线斜率"=w750, "二次多项式系数"=w748) -> (w746:T28)
                    n456 = global write "总磷断电保存全局变量.vi" "总磷仪器参数"(w746) -> ()
                  }
                }
              }
              frame Error {
              }
            }
            n457 = call "公式发生改变存储 (子VI).vi"("公式"=w725, "量程下拉列表输入"=w722, "测量模式下拉列表输入"=w723, "参数"=w724) -> ()  [unwired: 8 in]
            n458 = control-ref of="曲线模型"() -> (w720:refnum<vi>)
            n459 = control-ref of="量程下拉列表"() -> (w719:refnum<vi>)
            n460 = call "生成校准信息.vi"("table输入"="总磷", "量程下拉列表"=w719, "曲线模型"=w720) -> ()  [unwired: 9 in]
            n461 = One Button Dialog(message=w735) -> ()  [unwired: 1 in, 1 out]
          }
          frame "Center Button" {
            n462 = local read "曲线模型"() -> (w763:cluster{"X^2":dbl, "X":dbl, "B":dbl, "r^2":dbl})
            n463 = Unbundle By Name(w763) -> ("X^2"=w762:dbl, "X"=w760:dbl, "B"=w761:dbl)
            n464 = Build Array(w762, w760, w761) -> (w759:dbl[])
            n465 = Array To Cluster(array=w759) -> (cluster=w758:cluster{"[0]":dbl, "[1]":dbl, "[2]":dbl})
            n466 = local write "公式"(w758) -> ()
            n467 = call "公式复合写入.vi"("公式"=w758) -> ()  [unwired: 11 in]
            n468 = call "公式发生改变存储 (子VI).vi"("公式"=w758, "量程下拉列表输入"=w756, "测量模式下拉列表输入"=w755, "参数"=w757) -> ()  [unwired: 8 in]
            n469 = control-ref of="曲线模型"() -> (w753:refnum<vi>)
            n470 = control-ref of="量程下拉列表"() -> (w752:refnum<vi>)
            n471 = call "生成校准信息.vi"("table输入"="总磷", "量程下拉列表"=w752, "曲线模型"=w753) -> ()  [unwired: 9 in]
          }
          frame "Right Button" {
          }
          frame "Window Close" {
          }
        }
      }
      event "量程切换阈值读取": Value Change {
        n472 = event-data() -> ()  [unwired: 1 in, 6 out]
        n473 = property class="Enum (严格)"(reference=w769) -> ("Value"=w768:enum16{"总磷", "总氮"})  [unwired: 1 in, 2 out]
        n474 = call "总磷总氮量程读取.vi"("测量参数"=w768) -> ("error out"=w764:errorcluster, "量程参数读取"=w766:T31)  [unwired: 9 in]
        n475 = property class="Clust (严格)"(reference=w767, "Value"=w766) -> ()  [unwired: 1 in, 2 out]
        n476 = case shown="错误" w764 {
          tunnel: ["读取成功" ("消息") "读取失败" ("消息")] -> w765
          frame No Error {
          }
          frame Error {
          }
        }
        n477 = One Button Dialog(message=w765) -> ()  [unwired: 1 in, 1 out]
      }
      event "量程切换阈值写入": Value Change {
        n478 = event-data() -> ()  [unwired: 1 in, 6 out]
        n479 = property class="Enum (严格)"(reference=w776) -> ("Value"=w775:enum16{"总磷", "总氮"})  [unwired: 1 in, 2 out]
        n480 = call "总磷总氮量程写入.vi"("量程参数写入"="量程参数读取", "测量参数"=w775) -> ("error out"=w773:errorcluster)  [unwired: 8 in]
        n481 = case shown="无错误" w773 {
          tunnel: ["写入成功" ("消息") "写入失败" ("消息")] -> w774
          frame No Error {
          }
          frame Error {
          }
        }
        n482 = One Button Dialog(message=w774) -> ()  [unwired: 1 in, 1 out]
      }
    }
  }
  n483 = while {
    tunnel: [w786] -> _
    shift-right: [w784] -> _
    shift-left: w7 -> [w783]
    tunnel: w4 -> [w780]
    stop <- FALSE stop-if-true
    n484 = global read "VAR总磷全局变量.vi" "配置文件 path"() -> (w779:path)
    n485 = Read from Text File(file (use dialog)=w779, error in=w780) -> (text=w784:string, error out=w781:errorcluster)  [unwired: 2 in, 2 out]
    n486 = Not Equal?(x=w784, y=w783) -> (x != y?=w782:bool)
    n487 = case shown="真" w782 {
      tunnel: [w788 w792] -> w786
      tunnel: w779 -> [_ w791]
      tunnel: w781 -> [w788 w790]
      frame False {
      }
      frame True {
        # "文件发生改变进行更新"
        n488 = call <vilib>:"Open Config Data.vi"("error in (no error)"=w790, "configuration file path"=w791) -> ("error out"=w796:errorcluster, "refnum"=w795:T15)  [unwired: 7 in, 1 out]
        n489 = vi-ref "总磷断电保存全局变量.vi"() -> (w789:refnum<vi>)
        n490 = call <userlib>:"Read Panel from INI__ogtk.vi"("error in (no error)"=w796, "VI ref"=w789, "refnum"=w795) -> ("error out"=w794:errorcluster, "refnum out"=w793:T15)  [unwired: 7 in]
        n491 = call <vilib>:"Close Config Data.vi"("error in (no error)"=w794, "refnum"=w793) -> ("error out"=w792:errorcluster)  [unwired: 8 in, 1 out]
      }
    }
    n492 = Wait (ms)(milliseconds to wait=u32 1000 ("等待时间（毫秒）")) -> ()  [unwired: 1 out]
  }
